vi "rs3_decode_streams2.vi"(0 "Stream profile array":T2(array[cluster])=[{"ID"=42, "Profile"=521622968, "fps"=25, "RS Stream"=0, "RS Format"=0, "index"=2, "width"=1920, "height"=1080, "ppx"=0.0, "ppy"=0.0, "fx"=0.0, "fy"=0.0, "model"=0}, {"ID"=41, "Profile"=521634232, "fps"=25, "RS Stream"=0, "RS Format"=0, "index"=1, "width"=1920, "height"=1080, "ppx"=0.0, "ppy"=0.0, "fx"=0.0, "fy"=0.0, "model"=0}, {"ID"=42, "Profile"=521608632, "fps"=25, "RS Stream"=0, "RS Format"=0, "index"=2, "width"=1920, "height"=1080, "ppx"=951.85925, "ppy"=556.0496, "fx"=1428.9095, "fy"=1428.9095, "model"=4}, {"ID"=41, "Profile"=521617080, "fps"=25, "RS Stream"=0, "RS Format"=0, "index"=1, "width"=1920, "height"=1080, "ppx"=951.85925, "ppy"=556.0496, "fx"=1428.9095, "fy"=1428.9095, "model"=4}, {"ID"=41, "Profile"=521619128, "fps"=15, "RS Stream"=0, "RS Format"=0, "index"=1, "width"=1920, "height"=1080, "ppx"=0.0, "ppy"=0.0, "fx"=0.0, "fy"=0.0, "model"=0}, {"ID"=42, "Profile"=521623224, "fps"=15, "RS Stream"=0, "RS Format"=0, "index"=2, "width"=1920, "height"=1080, "ppx"=0.0, "ppy"=0.0, "fx"=0.0, "fy"=0.0, "model"=0}, {"ID"=42, "Profile"=521628088, "fps"=15, "RS Stream"=0, "RS Format"=0, "index"=2, "width"=1920, "height"=1080, "ppx"=951.85925, "ppy"=556.0496, "fx"=1428.9095, "fy"=1428.9095, "model"=4}, {"ID"=41, "Profile"=521627576, "fps"=15, "RS Stream"=0, "RS Format"=0, "index"=1, "width"=1920, "height"=1080, "ppx"=951.85925, "ppy"=556.0496, "fx"=1428.9095, "fy"=1428.9095, "model"=4}, {"ID"=41, "Profile"=521612728, "fps"=30, "RS Stream"=0, "RS Format"=0, "index"=0, "width"=1280, "height"=720, "ppx"=634.5728, "ppy"=370.69974, "fx"=952.6064, "fy"=952.6064, "model"=4}, {"ID"=41, "Profile"=521610424, "fps"=30, "RS Stream"=0, "RS Format"=0, "index"=0, "width"=1280, "height"=720, "ppx"=0.0, "ppy"=0.0, "fx"=0.0, "fy"=0.0, "model"=0}, {"ID"=42, "Profile"=521615544, "fps"=30, "RS Stream"=0, "RS Format"=0, "index"=2, "width"=1280, "height"=720, "ppx"=634.5728, "ppy"=370.69974, "fx"=952.6064, "fy"=952.6064, "model"=4}, {"ID"=41, "Profile"=521320344, "fps"=30, "RS Stream"=0, "RS Format"=0, "index"=1, "width"=1280, "height"=720, "ppx"=634.5728, "ppy"=370.69974, "fx"=952.6064, "fy"=952.6064, "model"=4}, {"ID"=41, "Profile"=521614520, "fps"=30, "RS Stream"=0, "RS Format"=0, "index"=0, "width"=1280, "height"=720, "ppx"=634.5728, "ppy"=370.69974, "fx"=952.6064, "fy"=952.6064, "model"=4}, {"ID"=41, "Profile"=521605816, "fps"=30, "RS Stream"=0, "RS Format"=0, "index"=0, "width"=1280, "height"=720, "ppx"=634.5728, "ppy"=370.69974, "fx"=952.6064, "fy"=952.6064, "model"=4}, {"ID"=41, "Profile"=521607608, "fps"=30, "RS Stream"=0, "RS Format"=0, "index"=0, "width"=1280, "height"=720, "ppx"=634.5728, "ppy"=370.69974, "fx"=952.6064, "fy"=952.6064, "model"=4}, {"ID"=41, "Profile"=521605560, "fps"=30, "RS Stream"=0, "RS Format"=0, "index"=0, "width"=1280, "height"=720, "ppx"=634.5728, "ppy"=370.69974, "fx"=952.6064, "fy"=952.6064, "model"=4}, {"ID"=41, "Profile"=521609912, "fps"=15, "RS Stream"=0, "RS Format"=0, "index"=0, "width"=1280, "height"=720, "ppx"=634.5728, "ppy"=370.69974, "fx"=952.6064, "fy"=952.6064, "model"=4}, {"ID"=41, "Profile"=521606584, "fps"=15, "RS Stream"=0, "RS Format"=0, "index"=0, "width"=1280, "height"=720, "ppx"=0.0, "ppy"=0.0, "fx"=0.0, "fy"=0.0, "model"=0}, {"ID"=41, "Profile"=521310872, "fps"=15, "RS Stream"=0, "RS Format"=0, "index"=1, "width"=1280, "height"=720, "ppx"=634.5728, "ppy"=370.69974, "fx"=952.6064, "fy"=952.6064, "model"=4}, {"ID"=42, "Profile"=521616824, "fps"=15, "RS Stream"=0, "RS Format"=0, "index"=2, "width"=1280, "height"=720, "ppx"=634.5728, "ppy"=370.69974, "fx"=952.6064, "fy"=952.6064, "model"=4}, {"ID"=41, "Profile"=521604024, "fps"=15, "RS Stream"=0, "RS Format"=0, "index"=0, "width"=1280, "height"=720, "ppx"=634.5728, "ppy"=370.69974, "fx"=952.6064, "fy"=952.6064, "model"=4}, {"ID"=41, "Profile"=521612984, "fps"=15, "RS Stream"=0, "RS Format"=0, "index"=0, "width"=1280, "height"=720, "ppx"=634.5728, "ppy"=370.69974, "fx"=952.6064, "fy"=952.6064, "model"=4}, {"ID"=41, "Profile"=521610168, "fps"=15, "RS Stream"=0, "RS Format"=0, "index"=0, "width"=1280, "height"=720, "ppx"=634.5728, "ppy"=370.69974, "fx"=952.6064, "fy"=952.6064, "model"=4}, {"ID"=41, "Profile"=521604536, "fps"=15, "RS Stream"=0, "RS Format"=0, "index"=0, "width"=1280, "height"=720, "ppx"=634.5728, "ppy"=370.69974, "fx"=952.6064, "fy"=952.6064, "model"=4}, {"ID"=41, "Profile"=521617848, "fps"=6, "RS Stream"=0, "RS Format"=0, "index"=0, "width"=1280, "height"=720, "ppx"=634.5728, "ppy"=370.69974, "fx"=952.6064, "fy"=952.6064, "model"=4}, {"ID"=41, "Profile"=521613752, "fps"=6, "RS Stream"=0, "RS Format"=0, "index"=0, "width"=1280, "height"=720, "ppx"=0.0, "ppy"=0.0, "fx"=0.0, "fy"=0.0, "model"=0}, {"ID"=41, "Profile"=521320600, "fps"=6, "RS Stream"=0, "RS Format"=0, "index"=1, "width"=1280, "height"=720, "ppx"=634.5728, "ppy"=370.69974, "fx"=952.6064, "fy"=952.6064, "model"=4}, {"ID"=42, "Profile"=521608888, "fps"=6, "RS Stream"=0, "RS Format"=0, "index"=2, "width"=1280, "height"=720, "ppx"=634.5728, "ppy"=370.69974, "fx"=952.6064, "fy"=952.6064, "model"=4}, {"ID"=41, "Profile"=521613240, "fps"=6, "RS Stream"=0, "RS Format"=0, "index"=0, "width"=1280, "height"=720, "ppx"=634.5728, "ppy"=370.69974, "fx"=952.6064, "fy"=952.6064, "model"=4}, {"ID"=41, "Profile"=521611704, "fps"=6, "RS Stream"=0, "RS Format"=0, "index"=0, "width"=1280, "height"=720, "ppx"=634.5728, "ppy"=370.69974, "fx"=952.6064, "fy"=952.6064, "model"=4}, {"ID"=41, "Profile"=521601720, "fps"=6, "RS Stream"=0, "RS Format"=0, "index"=0, "width"=1280, "height"=720, "ppx"=634.5728, "ppy"=370.69974, "fx"=952.6064, "fy"=952.6064, "model"=4}, {"ID"=41, "Profile"=521617336, "fps"=6, "RS Stream"=0, "RS Format"=0, "index"=0, "width"=1280, "height"=720, "ppx"=634.5728, "ppy"=370.69974, "fx"=952.6064, "fy"=952.6064, "model"=4}, {"ID"=41, "Profile"=521622712, "fps"=25, "RS Stream"=0, "RS Format"=0, "index"=1, "width"=960, "height"=540, "ppx"=0.0, "ppy"=0.0, "fx"=0.0, "fy"=0.0, "model"=0}, {"ID"=42, "Profile"=521633976, "fps"=25, "RS Stream"=0, "RS Format"=0, "index"=2, "width"=960, "height"=540, "ppx"=0.0, "ppy"=0.0, "fx"=0.0, "fy"=0.0, "model"=0}, {"ID"=42, "Profile"=521624504, "fps"=15, "RS Stream"=0, "RS Format"=0, "index"=2, "width"=960, "height"=540, "ppx"=0.0, "ppy"=0.0, "fx"=0.0, "fy"=0.0, "model"=0}, {"ID"=41, "Profile"=521622456, "fps"=15, "RS Stream"=0, "RS Format"=0, "index"=1, "width"=960, "height"=540, "ppx"=0.0, "ppy"=0.0, "fx"=0.0, "fy"=0.0, "model"=0}, {"ID"=41, "Profile"=521352856, "fps"=90, "RS Stream"=0, "RS Format"=0, "index"=0, "width"=848, "height"=480, "ppx"=420.38187, "ppy"=247.13316, "fx"=635.0709, "fy"=635.0709, "model"=4}, {"ID"=41, "Profile"=521351320, "fps"=90, "RS Stream"=0, "RS Format"=0, "index"=0, "width"=848, "height"=480, "ppx"=0.0, "ppy"=0.0, "fx"=0.0, "fy"=0.0, "model"=0}, {"ID"=41, "Profile"=521306776, "fps"=90, "RS Stream"=0, "RS Format"=0, "index"=1, "width"=848, "height"=480, "ppx"=420.38187, "ppy"=247.13316, "fx"=635.0709, "fy"=635.0709, "model"=4}, {"ID"=42, "Profile"=521614776, "fps"=90, "RS Stream"=0, "RS Format"=0, "index"=2, "width"=848, "height"=480, "ppx"=420.38187, "ppy"=247.13316, "fx"=635.0709, "fy"=635.0709, "model"=4}, {"ID"=41, "Profile"=521353624, "fps"=90, "RS Stream"=0, "RS Format"=0, "index"=0, "width"=848, "height"=480, "ppx"=420.38187, "ppy"=247.13316, "fx"=635.0709, "fy"=635.0709, "model"=4}, {"ID"=41, "Profile"=521339544, "fps"=90, "RS Stream"=0, "RS Format"=0, "index"=0, "width"=848, "height"=480, "ppx"=420.38187, "ppy"=247.13316, "fx"=635.0709, "fy"=635.0709, "model"=4}, {"ID"=41, "Profile"=521353368, "fps"=90, "RS Stream"=0, "RS Format"=0, "index"=0, "width"=848, "height"=480, "ppx"=420.38187, "ppy"=247.13316, "fx"=635.0709, "fy"=635.0709, "model"=4}, {"ID"=41, "Profile"=521351064, "fps"=90, "RS Stream"=0, "RS Format"=0, "index"=0, "width"=848, "height"=480, "ppx"=420.38187, "ppy"=247.13316, "fx"=635.0709, "fy"=635.0709, "model"=4}, {"ID"=41, "Profile"=521342104, "fps"=60, "RS Stream"=0, "RS Format"=0, "index"=0, "width"=848, "height"=480, "ppx"=420.38187, "ppy"=247.13316, "fx"=635.0709, "fy"=635.0709, "model"=4}, {"ID"=41, "Profile"=521341848, "fps"=60, "RS Stream"=0, "RS Format"=0, "index"=0, "width"=848, "height"=480, "ppx"=0.0, "ppy"=0.0, "fx"=0.0, "fy"=0.0, "model"=0}, {"ID"=42, "Profile"=521611960, "fps"=60, "RS Stream"=0, "RS Format"=0, "index"=2, "width"=848, "height"=480, "ppx"=420.38187, "ppy"=247.13316, "fx"=635.0709, "fy"=635.0709, "model"=4}, {"ID"=41, "Profile"=521310360, "fps"=60, "RS Stream"=0, "RS Format"=0, "index"=1, "width"=848, "height"=480, "ppx"=420.38187, "ppy"=247.13316, "fx"=635.0709, "fy"=635.0709, "model"=4}, {"ID"=41, "Profile"=521343384, "fps"=60, "RS Stream"=0, "RS Format"=0, "index"=0, "width"=848, "height"=480, "ppx"=420.38187, "ppy"=247.13316, "fx"=635.0709, "fy"=635.0709, "model"=4}, {"ID"=41, "Profile"=521342360, "fps"=60, "RS Stream"=0, "RS Format"=0, "index"=0, "width"=848, "height"=480, "ppx"=420.38187, "ppy"=247.13316, "fx"=635.0709, "fy"=635.0709, "model"=4}, {"ID"=41, "Profile"=521342616, "fps"=60, "RS Stream"=0, "RS Format"=0, "index"=0, "width"=848, "height"=480, "ppx"=420.38187, "ppy"=247.13316, "fx"=635.0709, "fy"=635.0709, "model"=4}, {"ID"=41, "Profile"=521354136, "fps"=60, "RS Stream"=0, "RS Format"=0, "index"=0, "width"=848, "height"=480, "ppx"=420.38187, "ppy"=247.13316, "fx"=635.0709, "fy"=635.0709, "model"=4}, {"ID"=41, "Profile"=521616056, "fps"=30, "RS Stream"=0, "RS Format"=0, "index"=0, "width"=848, "height"=480, "ppx"=420.38187, "ppy"=247.13316, "fx"=635.0709, "fy"=635.0709, "model"=4}, {"ID"=41, "Profile"=514733800, "fps"=30, "RS Stream"=0, "RS Format"=0, "index"=0, "width"=848, "height"=480, "ppx"=0.0, "ppy"=0.0, "fx"=0.0, "fy"=0.0, "model"=0}, {"ID"=42, "Profile"=521609144, "fps"=30, "RS Stream"=0, "RS Format"=0, "index"=2, "width"=848, "height"=480, "ppx"=420.38187, "ppy"=247.13316, "fx"=635.0709, "fy"=635.0709, "model"=4}, {"ID"=41, "Profile"=521310616, "fps"=30, "RS Stream"=0, "RS Format"=0, "index"=1, "width"=848, "height"=480, "ppx"=420.38187, "ppy"=247.13316, "fx"=635.0709, "fy"=635.0709, "model"=4}, {"ID"=41, "Profile"=521606840, "fps"=30, "RS Stream"=0, "RS Format"=0, "index"=0, "width"=848, "height"=480, "ppx"=420.38187, "ppy"=247.13316, "fx"=635.0709, "fy"=635.0709, "model"=4}, {"ID"=41, "Profile"=521603256, "fps"=30, "RS Stream"=0, "RS Format"=0, "index"=0, "width"=848, "height"=480, "ppx"=420.38187, "ppy"=247.13316, "fx"=635.0709, "fy"=635.0709, "model"=4}, {"ID"=41, "Profile"=521612472, "fps"=30, "RS Stream"=0, "RS Format"=0, "index"=0, "width"=848, "height"=480, "ppx"=420.38187, "ppy"=247.13316, "fx"=635.0709, "fy"=635.0709, "model"=4}, {"ID"=41, "Profile"=521343640, "fps"=30, "RS Stream"=0, "RS Format"=0, "index"=0, "width"=848, "height"=480, "ppx"=420.38187, "ppy"=247.13316, "fx"=635.0709, "fy"=635.0709, "model"=4}, {"ID"=41, "Profile"=521609400, "fps"=15, "RS Stream"=0, "RS Format"=0, "index"=0, "width"=848, "height"=480, "ppx"=420.38187, "ppy"=247.13316, "fx"=635.0709, "fy"=635.0709, "model"=4}, {"ID"=41, "Profile"=521606328, "fps"=15, "RS Stream"=0, "RS Format"=0, "index"=0, "width"=848, "height"=480, "ppx"=0.0, "ppy"=0.0, "fx"=0.0, "fy"=0.0, "model"=0}, {"ID"=41, "Profile"=521317272, "fps"=15, "RS Stream"=0, "RS Format"=0, "index"=1, "width"=848, "height"=480, "ppx"=420.38187, "ppy"=247.13316, "fx"=635.0709, "fy"=635.0709, "model"=4}, {"ID"=42, "Profile"=521615288, "fps"=15, "RS Stream"=0, "RS Format"=0, "index"=2, "width"=848, "height"=480, "ppx"=420.38187, "ppy"=247.13316, "fx"=635.0709, "fy"=635.0709, "model"=4}, {"ID"=41, "Profile"=521603512, "fps"=15, "RS Stream"=0, "RS Format"=0, "index"=0, "width"=848, "height"=480, "ppx"=420.38187, "ppy"=247.13316, "fx"=635.0709, "fy"=635.0709, "model"=4}, {"ID"=41, "Profile"=521602744, "fps"=15, "RS Stream"=0, "RS Format"=0, "index"=0, "width"=848, "height"=480, "ppx"=420.38187, "ppy"=247.13316, "fx"=635.0709, "fy"=635.0709, "model"=4}, {"ID"=41, "Profile"=521607096, "fps"=15, "RS Stream"=0, "RS Format"=0, "index"=0, "width"=848, "height"=480, "ppx"=420.38187, "ppy"=247.13316, "fx"=635.0709, "fy"=635.0709, "model"=4}, {"ID"=41, "Profile"=521617592, "fps"=15, "RS Stream"=0, "RS Format"=0, "index"=0, "width"=848, "height"=480, "ppx"=420.38187, "ppy"=247.13316, "fx"=635.0709, "fy"=635.0709, "model"=4}, {"ID"=41, "Profile"=521603768, "fps"=6, "RS Stream"=0, "RS Format"=0, "index"=0, "width"=848, "height"=480, "ppx"=420.38187, "ppy"=247.13316, "fx"=635.0709, "fy"=635.0709, "model"=4}, {"ID"=41, "Profile"=521604280, "fps"=6, "RS Stream"=0, "RS Format"=0, "index"=0, "width"=848, "height"=480, "ppx"=0.0, "ppy"=0.0, "fx"=0.0, "fy"=0.0, "model"=0}, {"ID"=42, "Profile"=521616568, "fps"=6, "RS Stream"=0, "RS Format"=0, "index"=2, "width"=848, "height"=480, "ppx"=420.38187, "ppy"=247.13316, "fx"=635.0709, "fy"=635.0709, "model"=4}, {"ID"=41, "Profile"=521315992, "fps"=6, "RS Stream"=0, "RS Format"=0, "index"=1, "width"=848, "height"=480, "ppx"=420.38187, "ppy"=247.13316, "fx"=635.0709, "fy"=635.0709, "model"=4}, {"ID"=41, "Profile"=521607864, "fps"=6, "RS Stream"=0, "RS Format"=0, "index"=0, "width"=848, "height"=480, "ppx"=420.38187, "ppy"=247.13316, "fx"=635.0709, "fy"=635.0709, "model"=4}, {"ID"=41, "Profile"=521616312, "fps"=6, "RS Stream"=0, "RS Format"=0, "index"=0, "width"=848, "height"=480, "ppx"=420.38187, "ppy"=247.13316, "fx"=635.0709, "fy"=635.0709, "model"=4}, {"ID"=41, "Profile"=521615800, "fps"=6, "RS Stream"=0, "RS Format"=0, "index"=0, "width"=848, "height"=480, "ppx"=420.38187, "ppy"=247.13316, "fx"=635.0709, "fy"=635.0709, "model"=4}, {"ID"=41, "Profile"=521610680, "fps"=6, "RS Stream"=0, "RS Format"=0, "index"=0, "width"=848, "height"=480, "ppx"=420.38187, "ppy"=247.13316, "fx"=635.0709, "fy"=635.0709, "model"=4}, {"ID"=41, "Profile"=521348504, "fps"=90, "RS Stream"=0, "RS Format"=0, "index"=0, "width"=640, "height"=480, "ppx"=316.38187, "ppy"=247.13316, "fx"=635.0709, "fy"=635.0709, "model"=4}, {"ID"=41, "Profile"=521354904, "fps"=90, "RS Stream"=0, "RS Format"=0, "index"=0, "width"=640, "height"=480, "ppx"=0.0, "ppy"=0.0, "fx"=0.0, "fy"=0.0, "model"=0}, {"ID"=42, "Profile"=521605304, "fps"=90, "RS Stream"=0, "RS Format"=0, "index"=2, "width"=640, "height"=480, "ppx"=316.38187, "ppy"=247.13316, "fx"=635.0709, "fy"=635.0709, "model"=4}, {"ID"=41, "Profile"=521322648, "fps"=90, "RS Stream"=0, "RS Format"=0, "index"=1, "width"=640, "height"=480, "ppx"=316.38187, "ppy"=247.13316, "fx"=635.0709, "fy"=635.0709, "model"=4}, {"ID"=41, "Profile"=521340056, "fps"=90, "RS Stream"=0, "RS Format"=0, "index"=0, "width"=640, "height"=480, "ppx"=316.38187, "ppy"=247.13316, "fx"=635.0709, "fy"=635.0709, "model"=4}, {"ID"=41, "Profile"=521355672, "fps"=90, "RS Stream"=0, "RS Format"=0, "index"=0, "width"=640, "height"=480, "ppx"=316.38187, "ppy"=247.13316, "fx"=635.0709, "fy"=635.0709, "model"=4}, {"ID"=41, "Profile"=521352088, "fps"=90, "RS Stream"=0, "RS Format"=0, "index"=0, "width"=640, "height"=480, "ppx"=316.38187, "ppy"=247.13316, "fx"=635.0709, "fy"=635.0709, "model"=4}, {"ID"=41, "Profile"=521351576, "fps"=90, "RS Stream"=0, "RS Format"=0, "index"=0, "width"=640, "height"=480, "ppx"=316.38187, "ppy"=247.13316, "fx"=635.0709, "fy"=635.0709, "model"=4}, {"ID"=41, "Profile"=521352344, "fps"=60, "RS Stream"=0, "RS Format"=0, "index"=0, "width"=640, "height"=480, "ppx"=316.38187, "ppy"=247.13316, "fx"=635.0709, "fy"=635.0709, "model"=4}, {"ID"=41, "Profile"=521354648, "fps"=60, "RS Stream"=0, "RS Format"=0, "index"=0, "width"=640, "height"=480, "ppx"=0.0, "ppy"=0.0, "fx"=0.0, "fy"=0.0, "model"=0}, {"ID"=41, "Profile"=521320088, "fps"=60, "RS Stream"=0, "RS Format"=0, "index"=1, "width"=640, "height"=480, "ppx"=316.38187, "ppy"=247.13316, "fx"=635.0709, "fy"=635.0709, "model"=4}, {"ID"=42, "Profile"=521615032, "fps"=60, "RS Stream"=0, "RS Format"=0, "index"=2, "width"=640, "height"=480, "ppx"=316.38187, "ppy"=247.13316, "fx"=635.0709, "fy"=635.0709, "model"=4}, {"ID"=41, "Profile"=521340312, "fps"=60, "RS Stream"=0, "RS Format"=0, "index"=0, "width"=640, "height"=480, "ppx"=316.38187, "ppy"=247.13316, "fx"=635.0709, "fy"=635.0709, "model"=4}, {"ID"=41, "Profile"=521342872, "fps"=60, "RS Stream"=0, "RS Format"=0, "index"=0, "width"=640, "height"=480, "ppx"=316.38187, "ppy"=247.13316, "fx"=635.0709, "fy"=635.0709, "model"=4}, {"ID"=41, "Profile"=521346200, "fps"=60, "RS Stream"=0, "RS Format"=0, "index"=0, "width"=640, "height"=480, "ppx"=316.38187, "ppy"=247.13316, "fx"=635.0709, "fy"=635.0709, "model"=4}, {"ID"=41, "Profile"=521345944, "fps"=60, "RS Stream"=0, "RS Format"=0, "index"=0, "width"=640, "height"=480, "ppx"=316.38187, "ppy"=247.13316, "fx"=635.0709, "fy"=635.0709, "model"=4}, {"ID"=41, "Profile"=521344408, "fps"=30, "RS Stream"=0, "RS Format"=0, "index"=0, "width"=640, "height"=480, "ppx"=316.38187, "ppy"=247.13316, "fx"=635.0709, "fy"=635.0709, "model"=4}, {"ID"=41, "Profile"=521348248, "fps"=30, "RS Stream"=0, "RS Format"=0, "index"=0, "width"=640, "height"=480, "ppx"=0.0, "ppy"=0.0, "fx"=0.0, "fy"=0.0, "model"=0}, {"ID"=41, "Profile"=521309592, "fps"=30, "RS Stream"=0, "RS Format"=0, "index"=1, "width"=640, "height"=480, "ppx"=316.38187, "ppy"=247.13316, "fx"=635.0709, "fy"=635.0709, "model"=4}, {"ID"=42, "Profile"=521607352, "fps"=30, "RS Stream"=0, "RS Format"=0, "index"=2, "width"=640, "height"=480, "ppx"=316.38187, "ppy"=247.13316, "fx"=635.0709, "fy"=635.0709, "model"=4}, {"ID"=41, "Profile"=521352600, "fps"=30, "RS Stream"=0, "RS Format"=0, "index"=0, "width"=640, "height"=480, "ppx"=316.38187, "ppy"=247.13316, "fx"=635.0709, "fy"=635.0709, "model"=4}, {"ID"=41, "Profile"=521344664, "fps"=30, "RS Stream"=0, "RS Format"=0, "index"=0, "width"=640, "height"=480, "ppx"=316.38187, "ppy"=247.13316, "fx"=635.0709, "fy"=635.0709, "model"=4}, {"ID"=41, "Profile"=521344920, "fps"=30, "RS Stream"=0, "RS Format"=0, "index"=0, "width"=640, "height"=480, "ppx"=316.38187, "ppy"=247.13316, "fx"=635.0709, "fy"=635.0709, "model"=4}, {"ID"=41, "Profile"=521350296, "fps"=30, "RS Stream"=0, "RS Format"=0, "index"=0, "width"=640, "height"=480, "ppx"=316.38187, "ppy"=247.13316, "fx"=635.0709, "fy"=635.0709, "model"=4}, {"ID"=41, "Profile"=521355160, "fps"=15, "RS Stream"=0, "RS Format"=0, "index"=0, "width"=640, "height"=480, "ppx"=316.38187, "ppy"=247.13316, "fx"=635.0709, "fy"=635.0709, "model"=4}, {"ID"=41, "Profile"=521341592, "fps"=15, "RS Stream"=0, "RS Format"=0, "index"=0, "width"=640, "height"=480, "ppx"=0.0, "ppy"=0.0, "fx"=0.0, "fy"=0.0, "model"=0}, {"ID"=41, "Profile"=521321368, "fps"=15, "RS Stream"=0, "RS Format"=0, "index"=1, "width"=640, "height"=480, "ppx"=316.38187, "ppy"=247.13316, "fx"=635.0709, "fy"=635.0709, "model"=4}, {"ID"=42, "Profile"=521608120, "fps"=15, "RS Stream"=0, "RS Format"=0, "index"=2, "width"=640, "height"=480, "ppx"=316.38187, "ppy"=247.13316, "fx"=635.0709, "fy"=635.0709, "model"=4}, {"ID"=41, "Profile"=521346968, "fps"=15, "RS Stream"=0, "RS Format"=0, "index"=0, "width"=640, "height"=480, "ppx"=316.38187, "ppy"=247.13316, "fx"=635.0709, "fy"=635.0709, "model"=4}, {"ID"=41, "Profile"=521348760, "fps"=15, "RS Stream"=0, "RS Format"=0, "index"=0, "width"=640, "height"=480, "ppx"=316.38187, "ppy"=247.13316, "fx"=635.0709, "fy"=635.0709, "model"=4}, {"ID"=41, "Profile"=521339800, "fps"=15, "RS Stream"=0, "RS Format"=0, "index"=0, "width"=640, "height"=480, "ppx"=316.38187, "ppy"=247.13316, "fx"=635.0709, "fy"=635.0709, "model"=4}, {"ID"=41, "Profile"=521350808, "fps"=15, "RS Stream"=0, "RS Format"=0, "index"=0, "width"=640, "height"=480, "ppx"=316.38187, "ppy"=247.13316, "fx"=635.0709, "fy"=635.0709, "model"=4}, {"ID"=41, "Profile"=521349016, "fps"=6, "RS Stream"=0, "RS Format"=0, "index"=0, "width"=640, "height"=480, "ppx"=316.38187, "ppy"=247.13316, "fx"=635.0709, "fy"=635.0709, "model"=4}, {"ID"=41, "Profile"=521346456, "fps"=6, "RS Stream"=0, "RS Format"=0, "index"=0, "width"=640, "height"=480, "ppx"=0.0, "ppy"=0.0, "fx"=0.0, "fy"=0.0, "model"=0}, {"ID"=42, "Profile"=521608376, "fps"=6, "RS Stream"=0, "RS Format"=0, "index"=2, "width"=640, "height"=480, "ppx"=316.38187, "ppy"=247.13316, "fx"=635.0709, "fy"=635.0709, "model"=4}, {"ID"=41, "Profile"=521313176, "fps"=6, "RS Stream"=0, "RS Format"=0, "index"=1, "width"=640, "height"=480, "ppx"=316.38187, "ppy"=247.13316, "fx"=635.0709, "fy"=635.0709, "model"=4}, {"ID"=41, "Profile"=521343128, "fps"=6, "RS Stream"=0, "RS Format"=0, "index"=0, "width"=640, "height"=480, "ppx"=316.38187, "ppy"=247.13316, "fx"=635.0709, "fy"=635.0709, "model"=4}, {"ID"=41, "Profile"=521349528, "fps"=6, "RS Stream"=0, "RS Format"=0, "index"=0, "width"=640, "height"=480, "ppx"=316.38187, "ppy"=247.13316, "fx"=635.0709, "fy"=635.0709, "model"=4}, {"ID"=41, "Profile"=521355416, "fps"=6, "RS Stream"=0, "RS Format"=0, "index"=0, "width"=640, "height"=480, "ppx"=316.38187, "ppy"=247.13316, "fx"=635.0709, "fy"=635.0709, "model"=4}, {"ID"=41, "Profile"=521349272, "fps"=6, "RS Stream"=0, "RS Format"=0, "index"=0, "width"=640, "height"=480, "ppx"=316.38187, "ppy"=247.13316, "fx"=635.0709, "fy"=635.0709, "model"=4}, {"ID"=41, "Profile"=521330840, "fps"=90, "RS Stream"=0, "RS Format"=0, "index"=0, "width"=640, "height"=360, "ppx"=317.2864, "ppy"=185.34987, "fx"=476.3032, "fy"=476.3032, "model"=4}, {"ID"=41, "Profile"=521330584, "fps"=90, "RS Stream"=0, "RS Format"=0, "index"=0, "width"=640, "height"=360, "ppx"=0.0, "ppy"=0.0, "fx"=0.0, "fy"=0.0, "model"=0}, {"ID"=41, "Profile"=521318296, "fps"=90, "RS Stream"=0, "RS Format"=0, "index"=1, "width"=640, "height"=360, "ppx"=317.2864, "ppy"=185.34987, "fx"=476.3032, "fy"=476.3032, "model"=4}, {"ID"=42, "Profile"=521609656, "fps"=90, "RS Stream"=0, "RS Format"=0, "index"=2, "width"=640, "height"=360, "ppx"=317.2864, "ppy"=185.34987, "fx"=476.3032, "fy"=476.3032, "model"=4}, {"ID"=41, "Profile"=521332120, "fps"=90, "RS Stream"=0, "RS Format"=0, "index"=0, "width"=640, "height"=360, "ppx"=317.2864, "ppy"=185.34987, "fx"=476.3032, "fy"=476.3032, "model"=4}, {"ID"=41, "Profile"=521331608, "fps"=90, "RS Stream"=0, "RS Format"=0, "index"=0, "width"=640, "height"=360, "ppx"=317.2864, "ppy"=185.34987, "fx"=476.3032, "fy"=476.3032, "model"=4}, {"ID"=41, "Profile"=521331864, "fps"=90, "RS Stream"=0, "RS Format"=0, "index"=0, "width"=640, "height"=360, "ppx"=317.2864, "ppy"=185.34987, "fx"=476.3032, "fy"=476.3032, "model"=4}, {"ID"=41, "Profile"=521326744, "fps"=90, "RS Stream"=0, "RS Format"=0, "index"=0, "width"=640, "height"=360, "ppx"=317.2864, "ppy"=185.34987, "fx"=476.3032, "fy"=476.3032, "model"=4}, {"ID"=41, "Profile"=521333912, "fps"=60, "RS Stream"=0, "RS Format"=0, "index"=0, "width"=640, "height"=360, "ppx"=317.2864, "ppy"=185.34987, "fx"=476.3032, "fy"=476.3032, "model"=4}, {"ID"=41, "Profile"=521333144, "fps"=60, "RS Stream"=0, "RS Format"=0, "index"=0, "width"=640, "height"=360, "ppx"=0.0, "ppy"=0.0, "fx"=0.0, "fy"=0.0, "model"=0}, {"ID"=42, "Profile"=521606072, "fps"=60, "RS Stream"=0, "RS Format"=0, "index"=2, "width"=640, "height"=360, "ppx"=317.2864, "ppy"=185.34987, "fx"=476.3032, "fy"=476.3032, "model"=4}, {"ID"=41, "Profile"=521321112, "fps"=60, "RS Stream"=0, "RS Format"=0, "index"=1, "width"=640, "height"=360, "ppx"=317.2864, "ppy"=185.34987, "fx"=476.3032, "fy"=476.3032, "model"=4}, {"ID"=41, "Profile"=521340824, "fps"=60, "RS Stream"=0, "RS Format"=0, "index"=0, "width"=640, "height"=360, "ppx"=317.2864, "ppy"=185.34987, "fx"=476.3032, "fy"=476.3032, "model"=4}, {"ID"=41, "Profile"=521353880, "fps"=60, "RS Stream"=0, "RS Format"=0, "index"=0, "width"=640, "height"=360, "ppx"=317.2864, "ppy"=185.34987, "fx"=476.3032, "fy"=476.3032, "model"=4}, {"ID"=41, "Profile"=521350552, "fps"=60, "RS Stream"=0, "RS Format"=0, "index"=0, "width"=640, "height"=360, "ppx"=317.2864, "ppy"=185.34987, "fx"=476.3032, "fy"=476.3032, "model"=4}, {"ID"=41, "Profile"=521332888, "fps"=60, "RS Stream"=0, "RS Format"=0, "index"=0, "width"=640, "height"=360, "ppx"=317.2864, "ppy"=185.34987, "fx"=476.3032, "fy"=476.3032, "model"=4}, {"ID"=41, "Profile"=521347224, "fps"=30, "RS Stream"=0, "RS Format"=0, "index"=0, "width"=640, "height"=360, "ppx"=317.2864, "ppy"=185.34987, "fx"=476.3032, "fy"=476.3032, "model"=4}, {"ID"=41, "Profile"=521349784, "fps"=30, "RS Stream"=0, "RS Format"=0, "index"=0, "width"=640, "height"=360, "ppx"=0.0, "ppy"=0.0, "fx"=0.0, "fy"=0.0, "model"=0}, {"ID"=42, "Profile"=521604792, "fps"=30, "RS Stream"=0, "RS Format"=0, "index"=2, "width"=640, "height"=360, "ppx"=317.2864, "ppy"=185.34987, "fx"=476.3032, "fy"=476.3032, "model"=4}, {"ID"=41, "Profile"=521319064, "fps"=30, "RS Stream"=0, "RS Format"=0, "index"=1, "width"=640, "height"=360, "ppx"=317.2864, "ppy"=185.34987, "fx"=476.3032, "fy"=476.3032, "model"=4}, {"ID"=41, "Profile"=521351832, "fps"=30, "RS Stream"=0, "RS Format"=0, "index"=0, "width"=640, "height"=360, "ppx"=317.2864, "ppy"=185.34987, "fx"=476.3032, "fy"=476.3032, "model"=4}, {"ID"=41, "Profile"=521347480, "fps"=30, "RS Stream"=0, "RS Format"=0, "index"=0, "width"=640, "height"=360, "ppx"=317.2864, "ppy"=185.34987, "fx"=476.3032, "fy"=476.3032, "model"=4}, {"ID"=41, "Profile"=521350040, "fps"=30, "RS Stream"=0, "RS Format"=0, "index"=0, "width"=640, "height"=360, "ppx"=317.2864, "ppy"=185.34987, "fx"=476.3032, "fy"=476.3032, "model"=4}, {"ID"=41, "Profile"=521345432, "fps"=30, "RS Stream"=0, "RS Format"=0, "index"=0, "width"=640, "height"=360, "ppx"=317.2864, "ppy"=185.34987, "fx"=476.3032, "fy"=476.3032, "model"=4}, {"ID"=41, "Profile"=521343896, "fps"=15, "RS Stream"=0, "RS Format"=0, "index"=0, "width"=640, "height"=360, "ppx"=317.2864, "ppy"=185.34987, "fx"=476.3032, "fy"=476.3032, "model"=4}, {"ID"=41, "Profile"=521340568, "fps"=15, "RS Stream"=0, "RS Format"=0, "index"=0, "width"=640, "height"=360, "ppx"=0.0, "ppy"=0.0, "fx"=0.0, "fy"=0.0, "model"=0}, {"ID"=41, "Profile"=521319320, "fps"=15, "RS Stream"=0, "RS Format"=0, "index"=1, "width"=640, "height"=360, "ppx"=317.2864, "ppy"=185.34987, "fx"=476.3032, "fy"=476.3032, "model"=4}, {"ID"=42, "Profile"=521613496, "fps"=15, "RS Stream"=0, "RS Format"=0, "index"=2, "width"=640, "height"=360, "ppx"=317.2864, "ppy"=185.34987, "fx"=476.3032, "fy"=476.3032, "model"=4}, {"ID"=41, "Profile"=521347736, "fps"=15, "RS Stream"=0, "RS Format"=0, "index"=0, "width"=640, "height"=360, "ppx"=317.2864, "ppy"=185.34987, "fx"=476.3032, "fy"=476.3032, "model"=4}, {"ID"=41, "Profile"=521345176, "fps"=15, "RS Stream"=0, "RS Format"=0, "index"=0, "width"=640, "height"=360, "ppx"=317.2864, "ppy"=185.34987, "fx"=476.3032, "fy"=476.3032, "model"=4}, {"ID"=41, "Profile"=521345688, "fps"=15, "RS Stream"=0, "RS Format"=0, "index"=0, "width"=640, "height"=360, "ppx"=317.2864, "ppy"=185.34987, "fx"=476.3032, "fy"=476.3032, "model"=4}, {"ID"=41, "Profile"=521347992, "fps"=15, "RS Stream"=0, "RS Format"=0, "index"=0, "width"=640, "height"=360, "ppx"=317.2864, "ppy"=185.34987, "fx"=476.3032, "fy"=476.3032, "model"=4}, {"ID"=41, "Profile"=521354392, "fps"=6, "RS Stream"=0, "RS Format"=0, "index"=0, "width"=640, "height"=360, "ppx"=317.2864, "ppy"=185.34987, "fx"=476.3032, "fy"=476.3032, "model"=4}, {"ID"=41, "Profile"=521341080, "fps"=6, "RS Stream"=0, "RS Format"=0, "index"=0, "width"=640, "height"=360, "ppx"=0.0, "ppy"=0.0, "fx"=0.0, "fy"=0.0, "model"=0}, {"ID"=42, "Profile"=521611448, "fps"=6, "RS Stream"=0, "RS Format"=0, "index"=2, "width"=640, "height"=360, "ppx"=317.2864, "ppy"=185.34987, "fx"=476.3032, "fy"=476.3032, "model"=4}, {"ID"=41, "Profile"=521314200, "fps"=6, "RS Stream"=0, "RS Format"=0, "index"=1, "width"=640, "height"=360, "ppx"=317.2864, "ppy"=185.34987, "fx"=476.3032, "fy"=476.3032, "model"=4}, {"ID"=41, "Profile"=521341336, "fps"=6, "RS Stream"=0, "RS Format"=0, "index"=0, "width"=640, "height"=360, "ppx"=317.2864, "ppy"=185.34987, "fx"=476.3032, "fy"=476.3032, "model"=4}, {"ID"=41, "Profile"=521344152, "fps"=6, "RS Stream"=0, "RS Format"=0, "index"=0, "width"=640, "height"=360, "ppx"=317.2864, "ppy"=185.34987, "fx"=476.3032, "fy"=476.3032, "model"=4}, {"ID"=41, "Profile"=521346712, "fps"=6, "RS Stream"=0, "RS Format"=0, "index"=0, "width"=640, "height"=360, "ppx"=317.2864, "ppy"=185.34987, "fx"=476.3032, "fy"=476.3032, "model"=4}, {"ID"=41, "Profile"=521353112, "fps"=6, "RS Stream"=0, "RS Format"=0, "index"=0, "width"=640, "height"=360, "ppx"=317.2864, "ppy"=185.34987, "fx"=476.3032, "fy"=476.3032, "model"=4}, {"ID"=41, "Profile"=521325720, "fps"=90, "RS Stream"=0, "RS Format"=0, "index"=0, "width"=480, "height"=270, "ppx"=237.96481, "ppy"=139.0124, "fx"=357.2274, "fy"=357.2274, "model"=4}, {"ID"=41, "Profile"=521331096, "fps"=90, "RS Stream"=0, "RS Format"=0, "index"=0, "width"=480, "height"=270, "ppx"=0.0, "ppy"=0.0, "fx"=0.0, "fy"=0.0, "model"=0}, {"ID"=42, "Profile"=521612216, "fps"=90, "RS Stream"=0, "RS Format"=0, "index"=2, "width"=480, "height"=270, "ppx"=237.96481, "ppy"=139.0124, "fx"=357.2274, "fy"=357.2274, "model"=4}, {"ID"=41, "Profile"=521312152, "fps"=90, "RS Stream"=0, "RS Format"=0, "index"=1, "width"=480, "height"=270, "ppx"=237.96481, "ppy"=139.0124, "fx"=357.2274, "fy"=357.2274, "model"=4}, {"ID"=41, "Profile"=521327768, "fps"=90, "RS Stream"=0, "RS Format"=0, "index"=0, "width"=480, "height"=270, "ppx"=237.96481, "ppy"=139.0124, "fx"=357.2274, "fy"=357.2274, "model"=4}, {"ID"=41, "Profile"=521336472, "fps"=90, "RS Stream"=0, "RS Format"=0, "index"=0, "width"=480, "height"=270, "ppx"=237.96481, "ppy"=139.0124, "fx"=357.2274, "fy"=357.2274, "model"=4}, {"ID"=41, "Profile"=521336728, "fps"=90, "RS Stream"=0, "RS Format"=0, "index"=0, "width"=480, "height"=270, "ppx"=237.96481, "ppy"=139.0124, "fx"=357.2274, "fy"=357.2274, "model"=4}, {"ID"=41, "Profile"=521326232, "fps"=90, "RS Stream"=0, "RS Format"=0, "index"=0, "width"=480, "height"=270, "ppx"=237.96481, "ppy"=139.0124, "fx"=357.2274, "fy"=357.2274, "model"=4}, {"ID"=41, "Profile"=521336984, "fps"=60, "RS Stream"=0, "RS Format"=0, "index"=0, "width"=480, "height"=270, "ppx"=237.96481, "ppy"=139.0124, "fx"=357.2274, "fy"=357.2274, "model"=4}, {"ID"=41, "Profile"=521328024, "fps"=60, "RS Stream"=0, "RS Format"=0, "index"=0, "width"=480, "height"=270, "ppx"=0.0, "ppy"=0.0, "fx"=0.0, "fy"=0.0, "model"=0}, {"ID"=41, "Profile"=521322904, "fps"=60, "RS Stream"=0, "RS Format"=0, "index"=1, "width"=480, "height"=270, "ppx"=237.96481, "ppy"=139.0124, "fx"=357.2274, "fy"=357.2274, "model"=4}, {"ID"=42, "Profile"=521603000, "fps"=60, "RS Stream"=0, "RS Format"=0, "index"=2, "width"=480, "height"=270, "ppx"=237.96481, "ppy"=139.0124, "fx"=357.2274, "fy"=357.2274, "model"=4}, {"ID"=41, "Profile"=521338264, "fps"=60, "RS Stream"=0, "RS Format"=0, "index"=0, "width"=480, "height"=270, "ppx"=237.96481, "ppy"=139.0124, "fx"=357.2274, "fy"=357.2274, "model"=4}, {"ID"=41, "Profile"=521337752, "fps"=60, "RS Stream"=0, "RS Format"=0, "index"=0, "width"=480, "height"=270, "ppx"=237.96481, "ppy"=139.0124, "fx"=357.2274, "fy"=357.2274, "model"=4}, {"ID"=41, "Profile"=521323416, "fps"=60, "RS Stream"=0, "RS Format"=0, "index"=0, "width"=480, "height"=270, "ppx"=237.96481, "ppy"=139.0124, "fx"=357.2274, "fy"=357.2274, "model"=4}, {"ID"=41, "Profile"=521337496, "fps"=60, "RS Stream"=0, "RS Format"=0, "index"=0, "width"=480, "height"=270, "ppx"=237.96481, "ppy"=139.0124, "fx"=357.2274, "fy"=357.2274, "model"=4}, {"ID"=41, "Profile"=521329816, "fps"=30, "RS Stream"=0, "RS Format"=0, "index"=0, "width"=480, "height"=270, "ppx"=237.96481, "ppy"=139.0124, "fx"=357.2274, "fy"=357.2274, "model"=4}, {"ID"=41, "Profile"=521328280, "fps"=30, "RS Stream"=0, "RS Format"=0, "index"=0, "width"=480, "height"=270, "ppx"=0.0, "ppy"=0.0, "fx"=0.0, "fy"=0.0, "model"=0}, {"ID"=42, "Profile"=521605048, "fps"=30, "RS Stream"=0, "RS Format"=0, "index"=2, "width"=480, "height"=270, "ppx"=237.96481, "ppy"=139.0124, "fx"=357.2274, "fy"=357.2274, "model"=4}, {"ID"=41, "Profile"=521316504, "fps"=30, "RS Stream"=0, "RS Format"=0, "index"=1, "width"=480, "height"=270, "ppx"=237.96481, "ppy"=139.0124, "fx"=357.2274, "fy"=357.2274, "model"=4}, {"ID"=41, "Profile"=521325464, "fps"=30, "RS Stream"=0, "RS Format"=0, "index"=0, "width"=480, "height"=270, "ppx"=237.96481, "ppy"=139.0124, "fx"=357.2274, "fy"=357.2274, "model"=4}, {"ID"=41, "Profile"=521325976, "fps"=30, "RS Stream"=0, "RS Format"=0, "index"=0, "width"=480, "height"=270, "ppx"=237.96481, "ppy"=139.0124, "fx"=357.2274, "fy"=357.2274, "model"=4}, {"ID"=41, "Profile"=521338520, "fps"=30, "RS Stream"=0, "RS Format"=0, "index"=0, "width"=480, "height"=270, "ppx"=237.96481, "ppy"=139.0124, "fx"=357.2274, "fy"=357.2274, "model"=4}, {"ID"=41, "Profile"=521332632, "fps"=30, "RS Stream"=0, "RS Format"=0, "index"=0, "width"=480, "height"=270, "ppx"=237.96481, "ppy"=139.0124, "fx"=357.2274, "fy"=357.2274, "model"=4}, {"ID"=41, "Profile"=521330328, "fps"=15, "RS Stream"=0, "RS Format"=0, "index"=0, "width"=480, "height"=270, "ppx"=237.96481, "ppy"=139.0124, "fx"=357.2274, "fy"=357.2274, "model"=4}, {"ID"=41, "Profile"=521328536, "fps"=15, "RS Stream"=0, "RS Format"=0, "index"=0, "width"=480, "height"=270, "ppx"=0.0, "ppy"=0.0, "fx"=0.0, "fy"=0.0, "model"=0}, {"ID"=41, "Profile"=521318808, "fps"=15, "RS Stream"=0, "RS Format"=0, "index"=1, "width"=480, "height"=270, "ppx"=237.96481, "ppy"=139.0124, "fx"=357.2274, "fy"=357.2274, "model"=4}, {"ID"=42, "Profile"=521610936, "fps"=15, "RS Stream"=0, "RS Format"=0, "index"=2, "width"=480, "height"=270, "ppx"=237.96481, "ppy"=139.0124, "fx"=357.2274, "fy"=357.2274, "model"=4}, {"ID"=41, "Profile"=521324440, "fps"=15, "RS Stream"=0, "RS Format"=0, "index"=0, "width"=480, "height"=270, "ppx"=237.96481, "ppy"=139.0124, "fx"=357.2274, "fy"=357.2274, "model"=4}, {"ID"=41, "Profile"=521328792, "fps"=15, "RS Stream"=0, "RS Format"=0, "index"=0, "width"=480, "height"=270, "ppx"=237.96481, "ppy"=139.0124, "fx"=357.2274, "fy"=357.2274, "model"=4}, {"ID"=41, "Profile"=521324184, "fps"=15, "RS Stream"=0, "RS Format"=0, "index"=0, "width"=480, "height"=270, "ppx"=237.96481, "ppy"=139.0124, "fx"=357.2274, "fy"=357.2274, "model"=4}, {"ID"=41, "Profile"=521323672, "fps"=15, "RS Stream"=0, "RS Format"=0, "index"=0, "width"=480, "height"=270, "ppx"=237.96481, "ppy"=139.0124, "fx"=357.2274, "fy"=357.2274, "model"=4}, {"ID"=41, "Profile"=521331352, "fps"=6, "RS Stream"=0, "RS Format"=0, "index"=0, "width"=480, "height"=270, "ppx"=237.96481, "ppy"=139.0124, "fx"=357.2274, "fy"=357.2274, "model"=4}, {"ID"=41, "Profile"=521324696, "fps"=6, "RS Stream"=0, "RS Format"=0, "index"=0, "width"=480, "height"=270, "ppx"=0.0, "ppy"=0.0, "fx"=0.0, "fy"=0.0, "model"=0}, {"ID"=42, "Profile"=521602488, "fps"=6, "RS Stream"=0, "RS Format"=0, "index"=2, "width"=480, "height"=270, "ppx"=237.96481, "ppy"=139.0124, "fx"=357.2274, "fy"=357.2274, "model"=4}, {"ID"=41, "Profile"=521314968, "fps"=6, "RS Stream"=0, "RS Format"=0, "index"=1, "width"=480, "height"=270, "ppx"=237.96481, "ppy"=139.0124, "fx"=357.2274, "fy"=357.2274, "model"=4}, {"ID"=41, "Profile"=521330072, "fps"=6, "RS Stream"=0, "RS Format"=0, "index"=0, "width"=480, "height"=270, "ppx"=237.96481, "ppy"=139.0124, "fx"=357.2274, "fy"=357.2274, "model"=4}, {"ID"=41, "Profile"=521326488, "fps"=6, "RS Stream"=0, "RS Format"=0, "index"=0, "width"=480, "height"=270, "ppx"=237.96481, "ppy"=139.0124, "fx"=357.2274, "fy"=357.2274, "model"=4}, {"ID"=41, "Profile"=521329304, "fps"=6, "RS Stream"=0, "RS Format"=0, "index"=0, "width"=480, "height"=270, "ppx"=237.96481, "ppy"=139.0124, "fx"=357.2274, "fy"=357.2274, "model"=4}, {"ID"=41, "Profile"=521329048, "fps"=6, "RS Stream"=0, "RS Format"=0, "index"=0, "width"=480, "height"=270, "ppx"=237.96481, "ppy"=139.0124, "fx"=357.2274, "fy"=357.2274, "model"=4}, {"ID"=41, "Profile"=521307032, "fps"=90, "RS Stream"=0, "RS Format"=0, "index"=0, "width"=424, "height"=240, "ppx"=210.19093, "ppy"=123.56658, "fx"=317.53546, "fy"=317.53546, "model"=4}, {"ID"=41, "Profile"=521322136, "fps"=90, "RS Stream"=0, "RS Format"=0, "index"=0, "width"=424, "height"=240, "ppx"=0.0, "ppy"=0.0, "fx"=0.0, "fy"=0.0, "model"=0}, {"ID"=42, "Profile"=521601976, "fps"=90, "RS Stream"=0, "RS Format"=0, "index"=2, "width"=424, "height"=240, "ppx"=210.19093, "ppy"=123.56658, "fx"=317.53546, "fy"=317.53546, "model"=4}, {"ID"=41, "Profile"=521315736, "fps"=90, "RS Stream"=0, "RS Format"=0, "index"=1, "width"=424, "height"=240, "ppx"=210.19093, "ppy"=123.56658, "fx"=317.53546, "fy"=317.53546, "model"=4}, {"ID"=41, "Profile"=521338776, "fps"=90, "RS Stream"=0, "RS Format"=0, "index"=0, "width"=424, "height"=240, "ppx"=210.19093, "ppy"=123.56658, "fx"=317.53546, "fy"=317.53546, "model"=4}, {"ID"=41, "Profile"=521307288, "fps"=90, "RS Stream"=0, "RS Format"=0, "index"=0, "width"=424, "height"=240, "ppx"=210.19093, "ppy"=123.56658, "fx"=317.53546, "fy"=317.53546, "model"=4}, {"ID"=41, "Profile"=521307544, "fps"=90, "RS Stream"=0, "RS Format"=0, "index"=0, "width"=424, "height"=240, "ppx"=210.19093, "ppy"=123.56658, "fx"=317.53546, "fy"=317.53546, "model"=4}, {"ID"=41, "Profile"=521321624, "fps"=90, "RS Stream"=0, "RS Format"=0, "index"=0, "width"=424, "height"=240, "ppx"=210.19093, "ppy"=123.56658, "fx"=317.53546, "fy"=317.53546, "model"=4}, {"ID"=41, "Profile"=521323928, "fps"=60, "RS Stream"=0, "RS Format"=0, "index"=0, "width"=424, "height"=240, "ppx"=210.19093, "ppy"=123.56658, "fx"=317.53546, "fy"=317.53546, "model"=4}, {"ID"=41, "Profile"=521339032, "fps"=60, "RS Stream"=0, "RS Format"=0, "index"=0, "width"=424, "height"=240, "ppx"=0.0, "ppy"=0.0, "fx"=0.0, "fy"=0.0, "model"=0}, {"ID"=42, "Profile"=521614008, "fps"=60, "RS Stream"=0, "RS Format"=0, "index"=2, "width"=424, "height"=240, "ppx"=210.19093, "ppy"=123.56658, "fx"=317.53546, "fy"=317.53546, "model"=4}, {"ID"=41, "Profile"=521313688, "fps"=60, "RS Stream"=0, "RS Format"=0, "index"=1, "width"=424, "height"=240, "ppx"=210.19093, "ppy"=123.56658, "fx"=317.53546, "fy"=317.53546, "model"=4}, {"ID"=41, "Profile"=521335192, "fps"=60, "RS Stream"=0, "RS Format"=0, "index"=0, "width"=424, "height"=240, "ppx"=210.19093, "ppy"=123.56658, "fx"=317.53546, "fy"=317.53546, "model"=4}, {"ID"=41, "Profile"=521337240, "fps"=60, "RS Stream"=0, "RS Format"=0, "index"=0, "width"=424, "height"=240, "ppx"=210.19093, "ppy"=123.56658, "fx"=317.53546, "fy"=317.53546, "model"=4}, {"ID"=41, "Profile"=521334680, "fps"=60, "RS Stream"=0, "RS Format"=0, "index"=0, "width"=424, "height"=240, "ppx"=210.19093, "ppy"=123.56658, "fx"=317.53546, "fy"=317.53546, "model"=4}, {"ID"=41, "Profile"=521334936, "fps"=60, "RS Stream"=0, "RS Format"=0, "index"=0, "width"=424, "height"=240, "ppx"=210.19093, "ppy"=123.56658, "fx"=317.53546, "fy"=317.53546, "model"=4}, {"ID"=41, "Profile"=521324952, "fps"=30, "RS Stream"=0, "RS Format"=0, "index"=0, "width"=424, "height"=240, "ppx"=210.19093, "ppy"=123.56658, "fx"=317.53546, "fy"=317.53546, "model"=4}, {"ID"=41, "Profile"=521335448, "fps"=30, "RS Stream"=0, "RS Format"=0, "index"=0, "width"=424, "height"=240, "ppx"=0.0, "ppy"=0.0, "fx"=0.0, "fy"=0.0, "model"=0}, {"ID"=42, "Profile"=521614264, "fps"=30, "RS Stream"=0, "RS Format"=0, "index"=2, "width"=424, "height"=240, "ppx"=210.19093, "ppy"=123.56658, "fx"=317.53546, "fy"=317.53546, "model"=4}, {"ID"=41, "Profile"=521314712, "fps"=30, "RS Stream"=0, "RS Format"=0, "index"=1, "width"=424, "height"=240, "ppx"=210.19093, "ppy"=123.56658, "fx"=317.53546, "fy"=317.53546, "model"=4}, {"ID"=41, "Profile"=521335704, "fps"=30, "RS Stream"=0, "RS Format"=0, "index"=0, "width"=424, "height"=240, "ppx"=210.19093, "ppy"=123.56658, "fx"=317.53546, "fy"=317.53546, "model"=4}, {"ID"=41, "Profile"=521327000, "fps"=30, "RS Stream"=0, "RS Format"=0, "index"=0, "width"=424, "height"=240, "ppx"=210.19093, "ppy"=123.56658, "fx"=317.53546, "fy"=317.53546, "model"=4}, {"ID"=41, "Profile"=521333656, "fps"=30, "RS Stream"=0, "RS Format"=0, "index"=0, "width"=424, "height"=240, "ppx"=210.19093, "ppy"=123.56658, "fx"=317.53546, "fy"=317.53546, "model"=4}, {"ID"=41, "Profile"=521336216, "fps"=30, "RS Stream"=0, "RS Format"=0, "index"=0, "width"=424, "height"=240, "ppx"=210.19093, "ppy"=123.56658, "fx"=317.53546, "fy"=317.53546, "model"=4}, {"ID"=41, "Profile"=521332376, "fps"=15, "RS Stream"=0, "RS Format"=0, "index"=0, "width"=424, "height"=240, "ppx"=210.19093, "ppy"=123.56658, "fx"=317.53546, "fy"=317.53546, "model"=4}, {"ID"=41, "Profile"=521339288, "fps"=15, "RS Stream"=0, "RS Format"=0, "index"=0, "width"=424, "height"=240, "ppx"=0.0, "ppy"=0.0, "fx"=0.0, "fy"=0.0, "model"=0}, {"ID"=42, "Profile"=521611192, "fps"=15, "RS Stream"=0, "RS Format"=0, "index"=2, "width"=424, "height"=240, "ppx"=210.19093, "ppy"=123.56658, "fx"=317.53546, "fy"=317.53546, "model"=4}, {"ID"=41, "Profile"=521310104, "fps"=15, "RS Stream"=0, "RS Format"=0, "index"=1, "width"=424, "height"=240, "ppx"=210.19093, "ppy"=123.56658, "fx"=317.53546, "fy"=317.53546, "model"=4}, {"ID"=41, "Profile"=521325208, "fps"=15, "RS Stream"=0, "RS Format"=0, "index"=0, "width"=424, "height"=240, "ppx"=210.19093, "ppy"=123.56658, "fx"=317.53546, "fy"=317.53546, "model"=4}, {"ID"=41, "Profile"=521329560, "fps"=15, "RS Stream"=0, "RS Format"=0, "index"=0, "width"=424, "height"=240, "ppx"=210.19093, "ppy"=123.56658, "fx"=317.53546, "fy"=317.53546, "model"=4}, {"ID"=41, "Profile"=521338008, "fps"=15, "RS Stream"=0, "RS Format"=0, "index"=0, "width"=424, "height"=240, "ppx"=210.19093, "ppy"=123.56658, "fx"=317.53546, "fy"=317.53546, "model"=4}, {"ID"=41, "Profile"=521335960, "fps"=15, "RS Stream"=0, "RS Format"=0, "index"=0, "width"=424, "height"=240, "ppx"=210.19093, "ppy"=123.56658, "fx"=317.53546, "fy"=317.53546, "model"=4}, {"ID"=41, "Profile"=521333400, "fps"=6, "RS Stream"=0, "RS Format"=0, "index"=0, "width"=424, "height"=240, "ppx"=210.19093, "ppy"=123.56658, "fx"=317.53546, "fy"=317.53546, "model"=4}, {"ID"=41, "Profile"=521334168, "fps"=6, "RS Stream"=0, "RS Format"=0, "index"=0, "width"=424, "height"=240, "ppx"=0.0, "ppy"=0.0, "fx"=0.0, "fy"=0.0, "model"=0}, {"ID"=42, "Profile"=521602232, "fps"=6, "RS Stream"=0, "RS Format"=0, "index"=2, "width"=424, "height"=240, "ppx"=210.19093, "ppy"=123.56658, "fx"=317.53546, "fy"=317.53546, "model"=4}, {"ID"=41, "Profile"=521311384, "fps"=6, "RS Stream"=0, "RS Format"=0, "index"=1, "width"=424, "height"=240, "ppx"=210.19093, "ppy"=123.56658, "fx"=317.53546, "fy"=317.53546, "model"=4}, {"ID"=41, "Profile"=521334424, "fps"=6, "RS Stream"=0, "RS Format"=0, "index"=0, "width"=424, "height"=240, "ppx"=210.19093, "ppy"=123.56658, "fx"=317.53546, "fy"=317.53546, "model"=4}, {"ID"=41, "Profile"=521323160, "fps"=6, "RS Stream"=0, "RS Format"=0, "index"=0, "width"=424, "height"=240, "ppx"=210.19093, "ppy"=123.56658, "fx"=317.53546, "fy"=317.53546, "model"=4}, {"ID"=41, "Profile"=521327512, "fps"=6, "RS Stream"=0, "RS Format"=0, "index"=0, "width"=424, "height"=240, "ppx"=210.19093, "ppy"=123.56658, "fx"=317.53546, "fy"=317.53546, "model"=4}, {"ID"=41, "Profile"=521327256, "fps"=6, "RS Stream"=0, "RS Format"=0, "index"=0, "width"=424, "height"=240, "ppx"=210.19093, "ppy"=123.56658, "fx"=317.53546, "fy"=317.53546, "model"=4}, {"ID"=40, "Profile"=521312408, "fps"=30, "RS Stream"=0, "RS Format"=0, "index"=0, "width"=1280, "height"=720, "ppx"=634.5728, "ppy"=370.69974, "fx"=952.6064, "fy"=952.6064, "model"=4}, {"ID"=40, "Profile"=521319832, "fps"=30, "RS Stream"=0, "RS Format"=0, "index"=0, "width"=1280, "height"=720, "ppx"=634.5728, "ppy"=370.69974, "fx"=952.6064, "fy"=952.6064, "model"=4}, {"ID"=40, "Profile"=521309336, "fps"=15, "RS Stream"=0, "RS Format"=0, "index"=0, "width"=1280, "height"=720, "ppx"=634.5728, "ppy"=370.69974, "fx"=952.6064, "fy"=952.6064, "model"=4}, {"ID"=40, "Profile"=521316248, "fps"=15, "RS Stream"=0, "RS Format"=0, "index"=0, "width"=1280, "height"=720, "ppx"=634.5728, "ppy"=370.69974, "fx"=952.6064, "fy"=952.6064, "model"=4}, {"ID"=40, "Profile"=521309080, "fps"=6, "RS Stream"=0, "RS Format"=0, "index"=0, "width"=1280, "height"=720, "ppx"=634.5728, "ppy"=370.69974, "fx"=952.6064, "fy"=952.6064, "model"=4}, {"ID"=40, "Profile"=521315224, "fps"=6, "RS Stream"=0, "RS Format"=0, "index"=0, "width"=1280, "height"=720, "ppx"=634.5728, "ppy"=370.69974, "fx"=952.6064, "fy"=952.6064, "model"=4}, {"ID"=40, "Profile"=521317784, "fps"=90, "RS Stream"=0, "RS Format"=0, "index"=0, "width"=848, "height"=480, "ppx"=420.38187, "ppy"=247.13316, "fx"=635.0709, "fy"=635.0709, "model"=4}, {"ID"=40, "Profile"=521322392, "fps"=90, "RS Stream"=0, "RS Format"=0, "index"=0, "width"=848, "height"=480, "ppx"=420.38187, "ppy"=247.13316, "fx"=635.0709, "fy"=635.0709, "model"=4}, {"ID"=40, "Profile"=521321880, "fps"=60, "RS Stream"=0, "RS Format"=0, "index"=0, "width"=848, "height"=480, "ppx"=420.38187, "ppy"=247.13316, "fx"=635.0709, "fy"=635.0709, "model"=4}, {"ID"=40, "Profile"=521318040, "fps"=60, "RS Stream"=0, "RS Format"=0, "index"=0, "width"=848, "height"=480, "ppx"=420.38187, "ppy"=247.13316, "fx"=635.0709, "fy"=635.0709, "model"=4}, {"ID"=40, "Profile"=521312920, "fps"=30, "RS Stream"=0, "RS Format"=0, "index"=0, "width"=848, "height"=480, "ppx"=420.38187, "ppy"=247.13316, "fx"=635.0709, "fy"=635.0709, "model"=4}, {"ID"=40, "Profile"=521320856, "fps"=30, "RS Stream"=0, "RS Format"=0, "index"=0, "width"=848, "height"=480, "ppx"=420.38187, "ppy"=247.13316, "fx"=635.0709, "fy"=635.0709, "model"=4}, {"ID"=40, "Profile"=521319576, "fps"=15, "RS Stream"=0, "RS Format"=0, "index"=0, "width"=848, "height"=480, "ppx"=420.38187, "ppy"=247.13316, "fx"=635.0709, "fy"=635.0709, "model"=4}, {"ID"=40, "Profile"=521308056, "fps"=15, "RS Stream"=0, "RS Format"=0, "index"=0, "width"=848, "height"=480, "ppx"=420.38187, "ppy"=247.13316, "fx"=635.0709, "fy"=635.0709, "model"=4}, {"ID"=40, "Profile"=521312664, "fps"=6, "RS Stream"=0, "RS Format"=0, "index"=0, "width"=848, "height"=480, "ppx"=420.38187, "ppy"=247.13316, "fx"=635.0709, "fy"=635.0709, "model"=4}, {"ID"=40, "Profile"=521308824, "fps"=6, "RS Stream"=0, "RS Format"=0, "index"=0, "width"=848, "height"=480, "ppx"=420.38187, "ppy"=247.13316, "fx"=635.0709, "fy"=635.0709, "model"=4}, {"ID"=40, "Profile"=521308568, "fps"=90, "RS Stream"=0, "RS Format"=0, "index"=0, "width"=640, "height"=480, "ppx"=316.38187, "ppy"=247.13316, "fx"=635.0709, "fy"=635.0709, "model"=4}, {"ID"=40, "Profile"=521313432, "fps"=90, "RS Stream"=0, "RS Format"=0, "index"=0, "width"=640, "height"=480, "ppx"=316.38187, "ppy"=247.13316, "fx"=635.0709, "fy"=635.0709, "model"=4}, {"ID"=40, "Profile"=521315480, "fps"=60, "RS Stream"=0, "RS Format"=0, "index"=0, "width"=640, "height"=480, "ppx"=316.38187, "ppy"=247.13316, "fx"=635.0709, "fy"=635.0709, "model"=4}, {"ID"=40, "Profile"=521318552, "fps"=60, "RS Stream"=0, "RS Format"=0, "index"=0, "width"=640, "height"=480, "ppx"=316.38187, "ppy"=247.13316, "fx"=635.0709, "fy"=635.0709, "model"=4}, {"ID"=40, "Profile"=521311128, "fps"=30, "RS Stream"=0, "RS Format"=0, "index"=0, "width"=640, "height"=480, "ppx"=316.38187, "ppy"=247.13316, "fx"=635.0709, "fy"=635.0709, "model"=4}, {"ID"=40, "Profile"=521309848, "fps"=30, "RS Stream"=0, "RS Format"=0, "index"=0, "width"=640, "height"=480, "ppx"=316.38187, "ppy"=247.13316, "fx"=635.0709, "fy"=635.0709, "model"=4}, {"ID"=40, "Profile"=521317528, "fps"=15, "RS Stream"=0, "RS Format"=0, "index"=0, "width"=640, "height"=480, "ppx"=316.38187, "ppy"=247.13316, "fx"=635.0709, "fy"=635.0709, "model"=4}, {"ID"=40, "Profile"=521316760, "fps"=15, "RS Stream"=0, "RS Format"=0, "index"=0, "width"=640, "height"=480, "ppx"=316.38187, "ppy"=247.13316, "fx"=635.0709, "fy"=635.0709, "model"=4}, {"ID"=40, "Profile"=521311896, "fps"=6, "RS Stream"=0, "RS Format"=0, "index"=0, "width"=640, "height"=480, "ppx"=316.38187, "ppy"=247.13316, "fx"=635.0709, "fy"=635.0709, "model"=4}, {"ID"=40, "Profile"=521307800, "fps"=6, "RS Stream"=0, "RS Format"=0, "index"=0, "width"=640, "height"=480, "ppx"=316.38187, "ppy"=247.13316, "fx"=635.0709, "fy"=635.0709, "model"=4}, {"ID"=40, "Profile"=521290648, "fps"=90, "RS Stream"=0, "RS Format"=0, "index"=0, "width"=640, "height"=360, "ppx"=317.2864, "ppy"=185.34987, "fx"=476.3032, "fy"=476.3032, "model"=4}, {"ID"=40, "Profile"=521306520, "fps"=90, "RS Stream"=0, "RS Format"=0, "index"=0, "width"=640, "height"=360, "ppx"=317.2864, "ppy"=185.34987, "fx"=476.3032, "fy"=476.3032, "model"=4}, {"ID"=40, "Profile"=521293208, "fps"=60, "RS Stream"=0, "RS Format"=0, "index"=0, "width"=640, "height"=360, "ppx"=317.2864, "ppy"=185.34987, "fx"=476.3032, "fy"=476.3032, "model"=4}, {"ID"=40, "Profile"=521292952, "fps"=60, "RS Stream"=0, "RS Format"=0, "index"=0, "width"=640, "height"=360, "ppx"=317.2864, "ppy"=185.34987, "fx"=476.3032, "fy"=476.3032, "model"=4}, {"ID"=40, "Profile"=521294232, "fps"=30, "RS Stream"=0, "RS Format"=0, "index"=0, "width"=640, "height"=360, "ppx"=317.2864, "ppy"=185.34987, "fx"=476.3032, "fy"=476.3032, "model"=4}, {"ID"=40, "Profile"=521293720, "fps"=30, "RS Stream"=0, "RS Format"=0, "index"=0, "width"=640, "height"=360, "ppx"=317.2864, "ppy"=185.34987, "fx"=476.3032, "fy"=476.3032, "model"=4}, {"ID"=40, "Profile"=521317016, "fps"=15, "RS Stream"=0, "RS Format"=0, "index"=0, "width"=640, "height"=360, "ppx"=317.2864, "ppy"=185.34987, "fx"=476.3032, "fy"=476.3032, "model"=4}, {"ID"=40, "Profile"=521308312, "fps"=15, "RS Stream"=0, "RS Format"=0, "index"=0, "width"=640, "height"=360, "ppx"=317.2864, "ppy"=185.34987, "fx"=476.3032, "fy"=476.3032, "model"=4}, {"ID"=40, "Profile"=521311640, "fps"=6, "RS Stream"=0, "RS Format"=0, "index"=0, "width"=640, "height"=360, "ppx"=317.2864, "ppy"=185.34987, "fx"=476.3032, "fy"=476.3032, "model"=4}, {"ID"=40, "Profile"=521313944, "fps"=6, "RS Stream"=0, "RS Format"=0, "index"=0, "width"=640, "height"=360, "ppx"=317.2864, "ppy"=185.34987, "fx"=476.3032, "fy"=476.3032, "model"=4}, {"ID"=40, "Profile"=521293464, "fps"=90, "RS Stream"=0, "RS Format"=0, "index"=0, "width"=480, "height"=270, "ppx"=237.96481, "ppy"=139.0124, "fx"=357.2274, "fy"=357.2274, "model"=4}, {"ID"=40, "Profile"=521297560, "fps"=90, "RS Stream"=0, "RS Format"=0, "index"=0, "width"=480, "height"=270, "ppx"=237.96481, "ppy"=139.0124, "fx"=357.2274, "fy"=357.2274, "model"=4}, {"ID"=40, "Profile"=521302680, "fps"=60, "RS Stream"=0, "RS Format"=0, "index"=0, "width"=480, "height"=270, "ppx"=237.96481, "ppy"=139.0124, "fx"=357.2274, "fy"=357.2274, "model"=4}, {"ID"=40, "Profile"=521300376, "fps"=60, "RS Stream"=0, "RS Format"=0, "index"=0, "width"=480, "height"=270, "ppx"=237.96481, "ppy"=139.0124, "fx"=357.2274, "fy"=357.2274, "model"=4}, {"ID"=40, "Profile"=521302936, "fps"=30, "RS Stream"=0, "RS Format"=0, "index"=0, "width"=480, "height"=270, "ppx"=237.96481, "ppy"=139.0124, "fx"=357.2274, "fy"=357.2274, "model"=4}, {"ID"=40, "Profile"=521301144, "fps"=30, "RS Stream"=0, "RS Format"=0, "index"=0, "width"=480, "height"=270, "ppx"=237.96481, "ppy"=139.0124, "fx"=357.2274, "fy"=357.2274, "model"=4}, {"ID"=40, "Profile"=521303192, "fps"=15, "RS Stream"=0, "RS Format"=0, "index"=0, "width"=480, "height"=270, "ppx"=237.96481, "ppy"=139.0124, "fx"=357.2274, "fy"=357.2274, "model"=4}, {"ID"=40, "Profile"=521304984, "fps"=15, "RS Stream"=0, "RS Format"=0, "index"=0, "width"=480, "height"=270, "ppx"=237.96481, "ppy"=139.0124, "fx"=357.2274, "fy"=357.2274, "model"=4}, {"ID"=40, "Profile"=521304216, "fps"=6, "RS Stream"=0, "RS Format"=0, "index"=0, "width"=480, "height"=270, "ppx"=237.96481, "ppy"=139.0124, "fx"=357.2274, "fy"=357.2274, "model"=4}, {"ID"=40, "Profile"=521303704, "fps"=6, "RS Stream"=0, "RS Format"=0, "index"=0, "width"=480, "height"=270, "ppx"=237.96481, "ppy"=139.0124, "fx"=357.2274, "fy"=357.2274, "model"=4}, {"ID"=40, "Profile"=521306264, "fps"=90, "RS Stream"=0, "RS Format"=0, "index"=0, "width"=424, "height"=240, "ppx"=210.19093, "ppy"=123.56658, "fx"=317.53546, "fy"=317.53546, "model"=4}, {"ID"=40, "Profile"=521301912, "fps"=90, "RS Stream"=0, "RS Format"=0, "index"=0, "width"=424, "height"=240, "ppx"=210.19093, "ppy"=123.56658, "fx"=317.53546, "fy"=317.53546, "model"=4}, {"ID"=40, "Profile"=521292184, "fps"=60, "RS Stream"=0, "RS Format"=0, "index"=0, "width"=424, "height"=240, "ppx"=210.19093, "ppy"=123.56658, "fx"=317.53546, "fy"=317.53546, "model"=4}, {"ID"=40, "Profile"=521291928, "fps"=60, "RS Stream"=0, "RS Format"=0, "index"=0, "width"=424, "height"=240, "ppx"=210.19093, "ppy"=123.56658, "fx"=317.53546, "fy"=317.53546, "model"=4}, {"ID"=40, "Profile"=521296792, "fps"=30, "RS Stream"=0, "RS Format"=0, "index"=0, "width"=424, "height"=240, "ppx"=210.19093, "ppy"=123.56658, "fx"=317.53546, "fy"=317.53546, "model"=4}, {"ID"=40, "Profile"=521300120, "fps"=30, "RS Stream"=0, "RS Format"=0, "index"=0, "width"=424, "height"=240, "ppx"=210.19093, "ppy"=123.56658, "fx"=317.53546, "fy"=317.53546, "model"=4}, {"ID"=40, "Profile"=521300632, "fps"=15, "RS Stream"=0, "RS Format"=0, "index"=0, "width"=424, "height"=240, "ppx"=210.19093, "ppy"=123.56658, "fx"=317.53546, "fy"=317.53546, "model"=4}, {"ID"=40, "Profile"=521302424, "fps"=15, "RS Stream"=0, "RS Format"=0, "index"=0, "width"=424, "height"=240, "ppx"=210.19093, "ppy"=123.56658, "fx"=317.53546, "fy"=317.53546, "model"=4}, {"ID"=40, "Profile"=521300888, "fps"=6, "RS Stream"=0, "RS Format"=0, "index"=0, "width"=424, "height"=240, "ppx"=210.19093, "ppy"=123.56658, "fx"=317.53546, "fy"=317.53546, "model"=4}, {"ID"=40, "Profile"=521292696, "fps"=6, "RS Stream"=0, "RS Format"=0, "index"=0, "width"=424, "height"=240, "ppx"=210.19093, "ppy"=123.56658, "fx"=317.53546, "fy"=317.53546, "model"=4}] {"model" items=["RS_DISTORTION_NONE", "RS_DISTORTION_MODIFIED_BROWN_CONRADY", "RS_DISTORTION_INVERSE_BROWN_CONRADY", "RS_DISTORTION_FTHETA", "RS_DISTORTION_BROWN_CONRADY", "RS_DISTORTION_COUNT"]; "RS Stream" items=["    RS2_STREAM_ANY,", "    RS2_STREAM_DEPTH                            , /**< Native stream of depth data produced by RealSense device */", "    RS2_STREAM_COLOR                            , /**< Native stream of color data captured by RealSense device */", "    RS2_STREAM_INFRARED                         , /**< Native stream of infrared data captured by RealSense device */", "    RS2_STREAM_FISHEYE                          , /**< Native stream of fish-eye (wide) data captured from the dedicate motion camera */", "    RS2_STREAM_GYRO                             , /**< Native stream of gyroscope motion data produced by RealSense device */", "    RS2_STREAM_ACCEL                            , /**< Native stream of accelerometer motion data produced by RealSense device */", "    RS2_STREAM_GPIO                             , /**< Signals from external device connected through GPIO */", "    RS2_STREAM_POSE                             , /**< 6 Degrees of Freedom pose data, calculated by RealSense device */", "    RS2_STREAM_CONFIDENCE,", "    RS2_STREAM_COUNT"]}) -> (1 "RGB ext.":T1(array[cluster])=[{"width"=424, "height"=240, "fps"=6, "Profile"=521292696, "ppx"=210.19093, "ppy"=123.56658, "fx"=317.53546, "fy"=317.53546, "model"=4}, {"width"=424, "height"=240, "fps"=15, "Profile"=521302424, "ppx"=210.19093, "ppy"=123.56658, "fx"=317.53546, "fy"=317.53546, "model"=4}, {"width"=424, "height"=240, "fps"=30, "Profile"=521300120, "ppx"=210.19093, "ppy"=123.56658, "fx"=317.53546, "fy"=317.53546, "model"=4}, {"width"=424, "height"=240, "fps"=60, "Profile"=521291928, "ppx"=210.19093, "ppy"=123.56658, "fx"=317.53546, "fy"=317.53546, "model"=4}, {"width"=424, "height"=240, "fps"=90, "Profile"=521301912, "ppx"=210.19093, "ppy"=123.56658, "fx"=317.53546, "fy"=317.53546, "model"=4}, {"width"=480, "height"=270, "fps"=6, "Profile"=521303704, "ppx"=237.96481, "ppy"=139.0124, "fx"=357.2274, "fy"=357.2274, "model"=4}, {"width"=480, "height"=270, "fps"=15, "Profile"=521304984, "ppx"=237.96481, "ppy"=139.0124, "fx"=357.2274, "fy"=357.2274, "model"=4}, {"width"=480, "height"=270, "fps"=30, "Profile"=521301144, "ppx"=237.96481, "ppy"=139.0124, "fx"=357.2274, "fy"=357.2274, "model"=4}, {"width"=480, "height"=270, "fps"=60, "Profile"=521300376, "ppx"=237.96481, "ppy"=139.0124, "fx"=357.2274, "fy"=357.2274, "model"=4}, {"width"=480, "height"=270, "fps"=90, "Profile"=521297560, "ppx"=237.96481, "ppy"=139.0124, "fx"=357.2274, "fy"=357.2274, "model"=4}, {"width"=640, "height"=360, "fps"=6, "Profile"=521313944, "ppx"=317.2864, "ppy"=185.34987, "fx"=476.3032, "fy"=476.3032, "model"=4}, {"width"=640, "height"=360, "fps"=15, "Profile"=521308312, "ppx"=317.2864, "ppy"=185.34987, "fx"=476.3032, "fy"=476.3032, "model"=4}, {"width"=640, "height"=360, "fps"=30, "Profile"=521293720, "ppx"=317.2864, "ppy"=185.34987, "fx"=476.3032, "fy"=476.3032, "model"=4}, {"width"=640, "height"=360, "fps"=60, "Profile"=521292952, "ppx"=317.2864, "ppy"=185.34987, "fx"=476.3032, "fy"=476.3032, "model"=4}, {"width"=640, "height"=360, "fps"=90, "Profile"=521306520, "ppx"=317.2864, "ppy"=185.34987, "fx"=476.3032, "fy"=476.3032, "model"=4}, {"width"=640, "height"=480, "fps"=6, "Profile"=521307800, "ppx"=316.38187, "ppy"=247.13316, "fx"=635.0709, "fy"=635.0709, "model"=4}, {"width"=640, "height"=480, "fps"=15, "Profile"=521316760, "ppx"=316.38187, "ppy"=247.13316, "fx"=635.0709, "fy"=635.0709, "model"=4}, {"width"=640, "height"=480, "fps"=30, "Profile"=521309848, "ppx"=316.38187, "ppy"=247.13316, "fx"=635.0709, "fy"=635.0709, "model"=4}, {"width"=640, "height"=480, "fps"=60, "Profile"=521318552, "ppx"=316.38187, "ppy"=247.13316, "fx"=635.0709, "fy"=635.0709, "model"=4}, {"width"=640, "height"=480, "fps"=90, "Profile"=521313432, "ppx"=316.38187, "ppy"=247.13316, "fx"=635.0709, "fy"=635.0709, "model"=4}, {"width"=848, "height"=480, "fps"=6, "Profile"=521308824, "ppx"=420.38187, "ppy"=247.13316, "fx"=635.0709, "fy"=635.0709, "model"=4}, {"width"=848, "height"=480, "fps"=15, "Profile"=521308056, "ppx"=420.38187, "ppy"=247.13316, "fx"=635.0709, "fy"=635.0709, "model"=4}, {"width"=848, "height"=480, "fps"=30, "Profile"=521320856, "ppx"=420.38187, "ppy"=247.13316, "fx"=635.0709, "fy"=635.0709, "model"=4}, {"width"=848, "height"=480, "fps"=60, "Profile"=521318040, "ppx"=420.38187, "ppy"=247.13316, "fx"=635.0709, "fy"=635.0709, "model"=4}, {"width"=848, "height"=480, "fps"=90, "Profile"=521322392, "ppx"=420.38187, "ppy"=247.13316, "fx"=635.0709, "fy"=635.0709, "model"=4}, {"width"=1280, "height"=720, "fps"=6, "Profile"=521315224, "ppx"=634.5728, "ppy"=370.69974, "fx"=952.6064, "fy"=952.6064, "model"=4}, {"width"=1280, "height"=720, "fps"=15, "Profile"=521316248, "ppx"=634.5728, "ppy"=370.69974, "fx"=952.6064, "fy"=952.6064, "model"=4}, {"width"=1280, "height"=720, "fps"=30, "Profile"=521319832, "ppx"=634.5728, "ppy"=370.69974, "fx"=952.6064, "fy"=952.6064, "model"=4}], 3 "RGB ext.":string[](array[string])=["424 x 240 @6fps", "424 x 240 @15fps", "424 x 240 @30fps", "424 x 240 @60fps", "424 x 240 @90fps", "480 x 270 @6fps", "480 x 270 @15fps", "480 x 270 @30fps", "480 x 270 @60fps", "480 x 270 @90fps", "640 x 360 @6fps", "640 x 360 @15fps", "640 x 360 @30fps", "640 x 360 @60fps", "640 x 360 @90fps", "640 x 480 @6fps", "640 x 480 @15fps", "640 x 480 @30fps", "640 x 480 @60fps", "640 x 480 @90fps", "848 x 480 @6fps", "848 x 480 @15fps", "848 x 480 @30fps", "848 x 480 @60fps", "848 x 480 @90fps", "1280 x 720 @6fps", "1280 x 720 @15fps", "1280 x 720 @30fps"], 4 "Unrectified L IR":T1(array[cluster])=[{"width"=424, "height"=240, "fps"=6, "Profile"=521292696, "ppx"=210.19093, "ppy"=123.56658, "fx"=317.53546, "fy"=317.53546, "model"=4}, {"width"=424, "height"=240, "fps"=15, "Profile"=521302424, "ppx"=210.19093, "ppy"=123.56658, "fx"=317.53546, "fy"=317.53546, "model"=4}, {"width"=424, "height"=240, "fps"=30, "Profile"=521300120, "ppx"=210.19093, "ppy"=123.56658, "fx"=317.53546, "fy"=317.53546, "model"=4}, {"width"=424, "height"=240, "fps"=60, "Profile"=521291928, "ppx"=210.19093, "ppy"=123.56658, "fx"=317.53546, "fy"=317.53546, "model"=4}, {"width"=424, "height"=240, "fps"=90, "Profile"=521301912, "ppx"=210.19093, "ppy"=123.56658, "fx"=317.53546, "fy"=317.53546, "model"=4}, {"width"=480, "height"=270, "fps"=6, "Profile"=521303704, "ppx"=237.96481, "ppy"=139.0124, "fx"=357.2274, "fy"=357.2274, "model"=4}, {"width"=480, "height"=270, "fps"=15, "Profile"=521304984, "ppx"=237.96481, "ppy"=139.0124, "fx"=357.2274, "fy"=357.2274, "model"=4}, {"width"=480, "height"=270, "fps"=30, "Profile"=521301144, "ppx"=237.96481, "ppy"=139.0124, "fx"=357.2274, "fy"=357.2274, "model"=4}, {"width"=480, "height"=270, "fps"=60, "Profile"=521300376, "ppx"=237.96481, "ppy"=139.0124, "fx"=357.2274, "fy"=357.2274, "model"=4}, {"width"=480, "height"=270, "fps"=90, "Profile"=521297560, "ppx"=237.96481, "ppy"=139.0124, "fx"=357.2274, "fy"=357.2274, "model"=4}, {"width"=640, "height"=360, "fps"=6, "Profile"=521313944, "ppx"=317.2864, "ppy"=185.34987, "fx"=476.3032, "fy"=476.3032, "model"=4}, {"width"=640, "height"=360, "fps"=15, "Profile"=521308312, "ppx"=317.2864, "ppy"=185.34987, "fx"=476.3032, "fy"=476.3032, "model"=4}, {"width"=640, "height"=360, "fps"=30, "Profile"=521293720, "ppx"=317.2864, "ppy"=185.34987, "fx"=476.3032, "fy"=476.3032, "model"=4}, {"width"=640, "height"=360, "fps"=60, "Profile"=521292952, "ppx"=317.2864, "ppy"=185.34987, "fx"=476.3032, "fy"=476.3032, "model"=4}, {"width"=640, "height"=360, "fps"=90, "Profile"=521306520, "ppx"=317.2864, "ppy"=185.34987, "fx"=476.3032, "fy"=476.3032, "model"=4}, {"width"=640, "height"=480, "fps"=6, "Profile"=521307800, "ppx"=316.38187, "ppy"=247.13316, "fx"=635.0709, "fy"=635.0709, "model"=4}, {"width"=640, "height"=480, "fps"=15, "Profile"=521316760, "ppx"=316.38187, "ppy"=247.13316, "fx"=635.0709, "fy"=635.0709, "model"=4}, {"width"=640, "height"=480, "fps"=30, "Profile"=521309848, "ppx"=316.38187, "ppy"=247.13316, "fx"=635.0709, "fy"=635.0709, "model"=4}, {"width"=640, "height"=480, "fps"=60, "Profile"=521318552, "ppx"=316.38187, "ppy"=247.13316, "fx"=635.0709, "fy"=635.0709, "model"=4}, {"width"=640, "height"=480, "fps"=90, "Profile"=521313432, "ppx"=316.38187, "ppy"=247.13316, "fx"=635.0709, "fy"=635.0709, "model"=4}, {"width"=848, "height"=480, "fps"=6, "Profile"=521308824, "ppx"=420.38187, "ppy"=247.13316, "fx"=635.0709, "fy"=635.0709, "model"=4}, {"width"=848, "height"=480, "fps"=15, "Profile"=521308056, "ppx"=420.38187, "ppy"=247.13316, "fx"=635.0709, "fy"=635.0709, "model"=4}, {"width"=848, "height"=480, "fps"=30, "Profile"=521320856, "ppx"=420.38187, "ppy"=247.13316, "fx"=635.0709, "fy"=635.0709, "model"=4}, {"width"=848, "height"=480, "fps"=60, "Profile"=521318040, "ppx"=420.38187, "ppy"=247.13316, "fx"=635.0709, "fy"=635.0709, "model"=4}, {"width"=848, "height"=480, "fps"=90, "Profile"=521322392, "ppx"=420.38187, "ppy"=247.13316, "fx"=635.0709, "fy"=635.0709, "model"=4}, {"width"=1280, "height"=720, "fps"=6, "Profile"=521315224, "ppx"=634.5728, "ppy"=370.69974, "fx"=952.6064, "fy"=952.6064, "model"=4}, {"width"=1280, "height"=720, "fps"=15, "Profile"=521316248, "ppx"=634.5728, "ppy"=370.69974, "fx"=952.6064, "fy"=952.6064, "model"=4}, {"width"=1280, "height"=720, "fps"=30, "Profile"=521319832, "ppx"=634.5728, "ppy"=370.69974, "fx"=952.6064, "fy"=952.6064, "model"=4}], 5 "Unrectified L IR":string[](array[string])=["424 x 240 @6fps", "424 x 240 @15fps", "424 x 240 @30fps", "424 x 240 @60fps", "424 x 240 @90fps", "480 x 270 @6fps", "480 x 270 @15fps", "480 x 270 @30fps", "480 x 270 @60fps", "480 x 270 @90fps", "640 x 360 @6fps", "640 x 360 @15fps", "640 x 360 @30fps", "640 x 360 @60fps", "640 x 360 @90fps", "640 x 480 @6fps", "640 x 480 @15fps", "640 x 480 @30fps", "640 x 480 @60fps", "640 x 480 @90fps", "848 x 480 @6fps", "848 x 480 @15fps", "848 x 480 @30fps", "848 x 480 @60fps", "848 x 480 @90fps", "1280 x 720 @6fps", "1280 x 720 @15fps", "1280 x 720 @30fps"], 6 "IR Left Array":string[](array[string])=["424 x 240 @6fps", "424 x 240 @15fps", "424 x 240 @30fps", "424 x 240 @60fps", "424 x 240 @90fps", "480 x 270 @6fps", "480 x 270 @15fps", "480 x 270 @30fps", "480 x 270 @60fps", "480 x 270 @90fps", "640 x 360 @6fps", "640 x 360 @15fps", "640 x 360 @30fps", "640 x 360 @60fps", "640 x 360 @90fps", "640 x 480 @6fps", "640 x 480 @15fps", "640 x 480 @30fps", "640 x 480 @60fps", "640 x 480 @90fps", "848 x 480 @6fps", "848 x 480 @15fps", "848 x 480 @30fps", "848 x 480 @60fps", "848 x 480 @90fps", "1280 x 720 @6fps", "1280 x 720 @15fps", "1280 x 720 @30fps", "1920 x 1080 @15fps", "1920 x 1080 @25fps"], 7 "IR Right Array":string[](array[string])=["424 x 240 @6fps", "424 x 240 @15fps", "424 x 240 @30fps", "424 x 240 @60fps", "424 x 240 @90fps", "480 x 270 @6fps", "480 x 270 @15fps", "480 x 270 @30fps", "480 x 270 @60fps", "480 x 270 @90fps", "640 x 360 @6fps", "640 x 360 @15fps", "640 x 360 @30fps", "640 x 360 @60fps", "640 x 360 @90fps", "640 x 480 @6fps", "640 x 480 @15fps", "640 x 480 @30fps", "640 x 480 @60fps", "640 x 480 @90fps", "848 x 480 @6fps", "848 x 480 @15fps", "848 x 480 @30fps", "848 x 480 @60fps", "848 x 480 @90fps", "1280 x 720 @6fps", "1280 x 720 @15fps", "1280 x 720 @30fps", "1920 x 1080 @15fps", "1920 x 1080 @25fps"], 10 "Unrectified R IR":string[](array[string])=["424 x 240 @6fps", "424 x 240 @15fps", "424 x 240 @30fps", "424 x 240 @60fps", "424 x 240 @90fps", "480 x 270 @6fps", "480 x 270 @15fps", "480 x 270 @30fps", "480 x 270 @60fps", "480 x 270 @90fps", "640 x 360 @6fps", "640 x 360 @15fps", "640 x 360 @30fps", "640 x 360 @60fps", "640 x 360 @90fps", "640 x 480 @6fps", "640 x 480 @15fps", "640 x 480 @30fps", "640 x 480 @60fps", "640 x 480 @90fps", "848 x 480 @6fps", "848 x 480 @15fps", "848 x 480 @30fps", "848 x 480 @60fps", "848 x 480 @90fps", "1280 x 720 @6fps", "1280 x 720 @15fps", "1280 x 720 @30fps"], 11 "Unrectified R  IR":T1(array[cluster])=[{"width"=424, "height"=240, "fps"=6, "Profile"=521292696, "ppx"=210.19093, "ppy"=123.56658, "fx"=317.53546, "fy"=317.53546, "model"=4}, {"width"=424, "height"=240, "fps"=15, "Profile"=521302424, "ppx"=210.19093, "ppy"=123.56658, "fx"=317.53546, "fy"=317.53546, "model"=4}, {"width"=424, "height"=240, "fps"=30, "Profile"=521300120, "ppx"=210.19093, "ppy"=123.56658, "fx"=317.53546, "fy"=317.53546, "model"=4}, {"width"=424, "height"=240, "fps"=60, "Profile"=521291928, "ppx"=210.19093, "ppy"=123.56658, "fx"=317.53546, "fy"=317.53546, "model"=4}, {"width"=424, "height"=240, "fps"=90, "Profile"=521301912, "ppx"=210.19093, "ppy"=123.56658, "fx"=317.53546, "fy"=317.53546, "model"=4}, {"width"=480, "height"=270, "fps"=6, "Profile"=521303704, "ppx"=237.96481, "ppy"=139.0124, "fx"=357.2274, "fy"=357.2274, "model"=4}, {"width"=480, "height"=270, "fps"=15, "Profile"=521304984, "ppx"=237.96481, "ppy"=139.0124, "fx"=357.2274, "fy"=357.2274, "model"=4}, {"width"=480, "height"=270, "fps"=30, "Profile"=521301144, "ppx"=237.96481, "ppy"=139.0124, "fx"=357.2274, "fy"=357.2274, "model"=4}, {"width"=480, "height"=270, "fps"=60, "Profile"=521300376, "ppx"=237.96481, "ppy"=139.0124, "fx"=357.2274, "fy"=357.2274, "model"=4}, {"width"=480, "height"=270, "fps"=90, "Profile"=521297560, "ppx"=237.96481, "ppy"=139.0124, "fx"=357.2274, "fy"=357.2274, "model"=4}, {"width"=640, "height"=360, "fps"=6, "Profile"=521313944, "ppx"=317.2864, "ppy"=185.34987, "fx"=476.3032, "fy"=476.3032, "model"=4}, {"width"=640, "height"=360, "fps"=15, "Profile"=521308312, "ppx"=317.2864, "ppy"=185.34987, "fx"=476.3032, "fy"=476.3032, "model"=4}, {"width"=640, "height"=360, "fps"=30, "Profile"=521293720, "ppx"=317.2864, "ppy"=185.34987, "fx"=476.3032, "fy"=476.3032, "model"=4}, {"width"=640, "height"=360, "fps"=60, "Profile"=521292952, "ppx"=317.2864, "ppy"=185.34987, "fx"=476.3032, "fy"=476.3032, "model"=4}, {"width"=640, "height"=360, "fps"=90, "Profile"=521306520, "ppx"=317.2864, "ppy"=185.34987, "fx"=476.3032, "fy"=476.3032, "model"=4}, {"width"=640, "height"=480, "fps"=6, "Profile"=521307800, "ppx"=316.38187, "ppy"=247.13316, "fx"=635.0709, "fy"=635.0709, "model"=4}, {"width"=640, "height"=480, "fps"=15, "Profile"=521316760, "ppx"=316.38187, "ppy"=247.13316, "fx"=635.0709, "fy"=635.0709, "model"=4}, {"width"=640, "height"=480, "fps"=30, "Profile"=521309848, "ppx"=316.38187, "ppy"=247.13316, "fx"=635.0709, "fy"=635.0709, "model"=4}, {"width"=640, "height"=480, "fps"=60, "Profile"=521318552, "ppx"=316.38187, "ppy"=247.13316, "fx"=635.0709, "fy"=635.0709, "model"=4}, {"width"=640, "height"=480, "fps"=90, "Profile"=521313432, "ppx"=316.38187, "ppy"=247.13316, "fx"=635.0709, "fy"=635.0709, "model"=4}, {"width"=848, "height"=480, "fps"=6, "Profile"=521308824, "ppx"=420.38187, "ppy"=247.13316, "fx"=635.0709, "fy"=635.0709, "model"=4}, {"width"=848, "height"=480, "fps"=15, "Profile"=521308056, "ppx"=420.38187, "ppy"=247.13316, "fx"=635.0709, "fy"=635.0709, "model"=4}, {"width"=848, "height"=480, "fps"=30, "Profile"=521320856, "ppx"=420.38187, "ppy"=247.13316, "fx"=635.0709, "fy"=635.0709, "model"=4}, {"width"=848, "height"=480, "fps"=60, "Profile"=521318040, "ppx"=420.38187, "ppy"=247.13316, "fx"=635.0709, "fy"=635.0709, "model"=4}, {"width"=848, "height"=480, "fps"=90, "Profile"=521322392, "ppx"=420.38187, "ppy"=247.13316, "fx"=635.0709, "fy"=635.0709, "model"=4}, {"width"=1280, "height"=720, "fps"=6, "Profile"=521315224, "ppx"=634.5728, "ppy"=370.69974, "fx"=952.6064, "fy"=952.6064, "model"=4}, {"width"=1280, "height"=720, "fps"=15, "Profile"=521316248, "ppx"=634.5728, "ppy"=370.69974, "fx"=952.6064, "fy"=952.6064, "model"=4}, {"width"=1280, "height"=720, "fps"=30, "Profile"=521319832, "ppx"=634.5728, "ppy"=370.69974, "fx"=952.6064, "fy"=952.6064, "model"=4}], 12 "IR left":T1(array[cluster])=[{"width"=424, "height"=240, "fps"=6, "Profile"=521311384, "ppx"=210.19093, "ppy"=123.56658, "fx"=317.53546, "fy"=317.53546, "model"=4}, {"width"=424, "height"=240, "fps"=15, "Profile"=521310104, "ppx"=210.19093, "ppy"=123.56658, "fx"=317.53546, "fy"=317.53546, "model"=4}, {"width"=424, "height"=240, "fps"=30, "Profile"=521314712, "ppx"=210.19093, "ppy"=123.56658, "fx"=317.53546, "fy"=317.53546, "model"=4}, {"width"=424, "height"=240, "fps"=60, "Profile"=521313688, "ppx"=210.19093, "ppy"=123.56658, "fx"=317.53546, "fy"=317.53546, "model"=4}, {"width"=424, "height"=240, "fps"=90, "Profile"=521315736, "ppx"=210.19093, "ppy"=123.56658, "fx"=317.53546, "fy"=317.53546, "model"=4}, {"width"=480, "height"=270, "fps"=6, "Profile"=521314968, "ppx"=237.96481, "ppy"=139.0124, "fx"=357.2274, "fy"=357.2274, "model"=4}, {"width"=480, "height"=270, "fps"=15, "Profile"=521318808, "ppx"=237.96481, "ppy"=139.0124, "fx"=357.2274, "fy"=357.2274, "model"=4}, {"width"=480, "height"=270, "fps"=30, "Profile"=521316504, "ppx"=237.96481, "ppy"=139.0124, "fx"=357.2274, "fy"=357.2274, "model"=4}, {"width"=480, "height"=270, "fps"=60, "Profile"=521322904, "ppx"=237.96481, "ppy"=139.0124, "fx"=357.2274, "fy"=357.2274, "model"=4}, {"width"=480, "height"=270, "fps"=90, "Profile"=521312152, "ppx"=237.96481, "ppy"=139.0124, "fx"=357.2274, "fy"=357.2274, "model"=4}, {"width"=640, "height"=360, "fps"=6, "Profile"=521314200, "ppx"=317.2864, "ppy"=185.34987, "fx"=476.3032, "fy"=476.3032, "model"=4}, {"width"=640, "height"=360, "fps"=15, "Profile"=521319320, "ppx"=317.2864, "ppy"=185.34987, "fx"=476.3032, "fy"=476.3032, "model"=4}, {"width"=640, "height"=360, "fps"=30, "Profile"=521319064, "ppx"=317.2864, "ppy"=185.34987, "fx"=476.3032, "fy"=476.3032, "model"=4}, {"width"=640, "height"=360, "fps"=60, "Profile"=521321112, "ppx"=317.2864, "ppy"=185.34987, "fx"=476.3032, "fy"=476.3032, "model"=4}, {"width"=640, "height"=360, "fps"=90, "Profile"=521318296, "ppx"=317.2864, "ppy"=185.34987, "fx"=476.3032, "fy"=476.3032, "model"=4}, {"width"=640, "height"=480, "fps"=6, "Profile"=521313176, "ppx"=316.38187, "ppy"=247.13316, "fx"=635.0709, "fy"=635.0709, "model"=4}, {"width"=640, "height"=480, "fps"=15, "Profile"=521321368, "ppx"=316.38187, "ppy"=247.13316, "fx"=635.0709, "fy"=635.0709, "model"=4}, {"width"=640, "height"=480, "fps"=30, "Profile"=521309592, "ppx"=316.38187, "ppy"=247.13316, "fx"=635.0709, "fy"=635.0709, "model"=4}, {"width"=640, "height"=480, "fps"=60, "Profile"=521320088, "ppx"=316.38187, "ppy"=247.13316, "fx"=635.0709, "fy"=635.0709, "model"=4}, {"width"=640, "height"=480, "fps"=90, "Profile"=521322648, "ppx"=316.38187, "ppy"=247.13316, "fx"=635.0709, "fy"=635.0709, "model"=4}, {"width"=848, "height"=480, "fps"=6, "Profile"=521315992, "ppx"=420.38187, "ppy"=247.13316, "fx"=635.0709, "fy"=635.0709, "model"=4}, {"width"=848, "height"=480, "fps"=15, "Profile"=521317272, "ppx"=420.38187, "ppy"=247.13316, "fx"=635.0709, "fy"=635.0709, "model"=4}, {"width"=848, "height"=480, "fps"=30, "Profile"=521310616, "ppx"=420.38187, "ppy"=247.13316, "fx"=635.0709, "fy"=635.0709, "model"=4}, {"width"=848, "height"=480, "fps"=60, "Profile"=521310360, "ppx"=420.38187, "ppy"=247.13316, "fx"=635.0709, "fy"=635.0709, "model"=4}, {"width"=848, "height"=480, "fps"=90, "Profile"=521306776, "ppx"=420.38187, "ppy"=247.13316, "fx"=635.0709, "fy"=635.0709, "model"=4}, {"width"=1280, "height"=720, "fps"=6, "Profile"=521320600, "ppx"=634.5728, "ppy"=370.69974, "fx"=952.6064, "fy"=952.6064, "model"=4}, {"width"=1280, "height"=720, "fps"=15, "Profile"=521310872, "ppx"=634.5728, "ppy"=370.69974, "fx"=952.6064, "fy"=952.6064, "model"=4}, {"width"=1280, "height"=720, "fps"=30, "Profile"=521320344, "ppx"=634.5728, "ppy"=370.69974, "fx"=952.6064, "fy"=952.6064, "model"=4}, {"width"=1920, "height"=1080, "fps"=15, "Profile"=521627576, "ppx"=951.85925, "ppy"=556.0496, "fx"=1428.9095, "fy"=1428.9095, "model"=4}, {"width"=1920, "height"=1080, "fps"=25, "Profile"=521617080, "ppx"=951.85925, "ppy"=556.0496, "fx"=1428.9095, "fy"=1428.9095, "model"=4}], 13 "IR Right":T1(array[cluster])=[{"width"=424, "height"=240, "fps"=6, "Profile"=521602232, "ppx"=210.19093, "ppy"=123.56658, "fx"=317.53546, "fy"=317.53546, "model"=4}, {"width"=424, "height"=240, "fps"=15, "Profile"=521611192, "ppx"=210.19093, "ppy"=123.56658, "fx"=317.53546, "fy"=317.53546, "model"=4}, {"width"=424, "height"=240, "fps"=30, "Profile"=521614264, "ppx"=210.19093, "ppy"=123.56658, "fx"=317.53546, "fy"=317.53546, "model"=4}, {"width"=424, "height"=240, "fps"=60, "Profile"=521614008, "ppx"=210.19093, "ppy"=123.56658, "fx"=317.53546, "fy"=317.53546, "model"=4}, {"width"=424, "height"=240, "fps"=90, "Profile"=521601976, "ppx"=210.19093, "ppy"=123.56658, "fx"=317.53546, "fy"=317.53546, "model"=4}, {"width"=480, "height"=270, "fps"=6, "Profile"=521602488, "ppx"=237.96481, "ppy"=139.0124, "fx"=357.2274, "fy"=357.2274, "model"=4}, {"width"=480, "height"=270, "fps"=15, "Profile"=521610936, "ppx"=237.96481, "ppy"=139.0124, "fx"=357.2274, "fy"=357.2274, "model"=4}, {"width"=480, "height"=270, "fps"=30, "Profile"=521605048, "ppx"=237.96481, "ppy"=139.0124, "fx"=357.2274, "fy"=357.2274, "model"=4}, {"width"=480, "height"=270, "fps"=60, "Profile"=521603000, "ppx"=237.96481, "ppy"=139.0124, "fx"=357.2274, "fy"=357.2274, "model"=4}, {"width"=480, "height"=270, "fps"=90, "Profile"=521612216, "ppx"=237.96481, "ppy"=139.0124, "fx"=357.2274, "fy"=357.2274, "model"=4}, {"width"=640, "height"=360, "fps"=6, "Profile"=521611448, "ppx"=317.2864, "ppy"=185.34987, "fx"=476.3032, "fy"=476.3032, "model"=4}, {"width"=640, "height"=360, "fps"=15, "Profile"=521613496, "ppx"=317.2864, "ppy"=185.34987, "fx"=476.3032, "fy"=476.3032, "model"=4}, {"width"=640, "height"=360, "fps"=30, "Profile"=521604792, "ppx"=317.2864, "ppy"=185.34987, "fx"=476.3032, "fy"=476.3032, "model"=4}, {"width"=640, "height"=360, "fps"=60, "Profile"=521606072, "ppx"=317.2864, "ppy"=185.34987, "fx"=476.3032, "fy"=476.3032, "model"=4}, {"width"=640, "height"=360, "fps"=90, "Profile"=521609656, "ppx"=317.2864, "ppy"=185.34987, "fx"=476.3032, "fy"=476.3032, "model"=4}, {"width"=640, "height"=480, "fps"=6, "Profile"=521608376, "ppx"=316.38187, "ppy"=247.13316, "fx"=635.0709, "fy"=635.0709, "model"=4}, {"width"=640, "height"=480, "fps"=15, "Profile"=521608120, "ppx"=316.38187, "ppy"=247.13316, "fx"=635.0709, "fy"=635.0709, "model"=4}, {"width"=640, "height"=480, "fps"=30, "Profile"=521607352, "ppx"=316.38187, "ppy"=247.13316, "fx"=635.0709, "fy"=635.0709, "model"=4}, {"width"=640, "height"=480, "fps"=60, "Profile"=521615032, "ppx"=316.38187, "ppy"=247.13316, "fx"=635.0709, "fy"=635.0709, "model"=4}, {"width"=640, "height"=480, "fps"=90, "Profile"=521605304, "ppx"=316.38187, "ppy"=247.13316, "fx"=635.0709, "fy"=635.0709, "model"=4}, {"width"=848, "height"=480, "fps"=6, "Profile"=521616568, "ppx"=420.38187, "ppy"=247.13316, "fx"=635.0709, "fy"=635.0709, "model"=4}, {"width"=848, "height"=480, "fps"=15, "Profile"=521615288, "ppx"=420.38187, "ppy"=247.13316, "fx"=635.0709, "fy"=635.0709, "model"=4}, {"width"=848, "height"=480, "fps"=30, "Profile"=521609144, "ppx"=420.38187, "ppy"=247.13316, "fx"=635.0709, "fy"=635.0709, "model"=4}, {"width"=848, "height"=480, "fps"=60, "Profile"=521611960, "ppx"=420.38187, "ppy"=247.13316, "fx"=635.0709, "fy"=635.0709, "model"=4}, {"width"=848, "height"=480, "fps"=90, "Profile"=521614776, "ppx"=420.38187, "ppy"=247.13316, "fx"=635.0709, "fy"=635.0709, "model"=4}, {"width"=1280, "height"=720, "fps"=6, "Profile"=521608888, "ppx"=634.5728, "ppy"=370.69974, "fx"=952.6064, "fy"=952.6064, "model"=4}, {"width"=1280, "height"=720, "fps"=15, "Profile"=521616824, "ppx"=634.5728, "ppy"=370.69974, "fx"=952.6064, "fy"=952.6064, "model"=4}, {"width"=1280, "height"=720, "fps"=30, "Profile"=521615544, "ppx"=634.5728, "ppy"=370.69974, "fx"=952.6064, "fy"=952.6064, "model"=4}, {"width"=1920, "height"=1080, "fps"=15, "Profile"=521628088, "ppx"=951.85925, "ppy"=556.0496, "fx"=1428.9095, "fy"=1428.9095, "model"=4}, {"width"=1920, "height"=1080, "fps"=25, "Profile"=521608632, "ppx"=951.85925, "ppy"=556.0496, "fx"=1428.9095, "fy"=1428.9095, "model"=4}], 14 "Depth Stream":T1(array[cluster])=[{"width"=424, "height"=240, "fps"=6, "Profile"=521292696, "ppx"=210.19093, "ppy"=123.56658, "fx"=317.53546, "fy"=317.53546, "model"=4}, {"width"=424, "height"=240, "fps"=15, "Profile"=521302424, "ppx"=210.19093, "ppy"=123.56658, "fx"=317.53546, "fy"=317.53546, "model"=4}, {"width"=424, "height"=240, "fps"=30, "Profile"=521300120, "ppx"=210.19093, "ppy"=123.56658, "fx"=317.53546, "fy"=317.53546, "model"=4}, {"width"=424, "height"=240, "fps"=60, "Profile"=521291928, "ppx"=210.19093, "ppy"=123.56658, "fx"=317.53546, "fy"=317.53546, "model"=4}, {"width"=424, "height"=240, "fps"=90, "Profile"=521301912, "ppx"=210.19093, "ppy"=123.56658, "fx"=317.53546, "fy"=317.53546, "model"=4}, {"width"=480, "height"=270, "fps"=6, "Profile"=521303704, "ppx"=237.96481, "ppy"=139.0124, "fx"=357.2274, "fy"=357.2274, "model"=4}, {"width"=480, "height"=270, "fps"=15, "Profile"=521304984, "ppx"=237.96481, "ppy"=139.0124, "fx"=357.2274, "fy"=357.2274, "model"=4}, {"width"=480, "height"=270, "fps"=30, "Profile"=521301144, "ppx"=237.96481, "ppy"=139.0124, "fx"=357.2274, "fy"=357.2274, "model"=4}, {"width"=480, "height"=270, "fps"=60, "Profile"=521300376, "ppx"=237.96481, "ppy"=139.0124, "fx"=357.2274, "fy"=357.2274, "model"=4}, {"width"=480, "height"=270, "fps"=90, "Profile"=521297560, "ppx"=237.96481, "ppy"=139.0124, "fx"=357.2274, "fy"=357.2274, "model"=4}, {"width"=640, "height"=360, "fps"=6, "Profile"=521313944, "ppx"=317.2864, "ppy"=185.34987, "fx"=476.3032, "fy"=476.3032, "model"=4}, {"width"=640, "height"=360, "fps"=15, "Profile"=521308312, "ppx"=317.2864, "ppy"=185.34987, "fx"=476.3032, "fy"=476.3032, "model"=4}, {"width"=640, "height"=360, "fps"=30, "Profile"=521293720, "ppx"=317.2864, "ppy"=185.34987, "fx"=476.3032, "fy"=476.3032, "model"=4}, {"width"=640, "height"=360, "fps"=60, "Profile"=521292952, "ppx"=317.2864, "ppy"=185.34987, "fx"=476.3032, "fy"=476.3032, "model"=4}, {"width"=640, "height"=360, "fps"=90, "Profile"=521306520, "ppx"=317.2864, "ppy"=185.34987, "fx"=476.3032, "fy"=476.3032, "model"=4}, {"width"=640, "height"=480, "fps"=6, "Profile"=521307800, "ppx"=316.38187, "ppy"=247.13316, "fx"=635.0709, "fy"=635.0709, "model"=4}, {"width"=640, "height"=480, "fps"=15, "Profile"=521316760, "ppx"=316.38187, "ppy"=247.13316, "fx"=635.0709, "fy"=635.0709, "model"=4}, {"width"=640, "height"=480, "fps"=30, "Profile"=521309848, "ppx"=316.38187, "ppy"=247.13316, "fx"=635.0709, "fy"=635.0709, "model"=4}, {"width"=640, "height"=480, "fps"=60, "Profile"=521318552, "ppx"=316.38187, "ppy"=247.13316, "fx"=635.0709, "fy"=635.0709, "model"=4}, {"width"=640, "height"=480, "fps"=90, "Profile"=521313432, "ppx"=316.38187, "ppy"=247.13316, "fx"=635.0709, "fy"=635.0709, "model"=4}, {"width"=848, "height"=480, "fps"=6, "Profile"=521308824, "ppx"=420.38187, "ppy"=247.13316, "fx"=635.0709, "fy"=635.0709, "model"=4}, {"width"=848, "height"=480, "fps"=15, "Profile"=521308056, "ppx"=420.38187, "ppy"=247.13316, "fx"=635.0709, "fy"=635.0709, "model"=4}, {"width"=848, "height"=480, "fps"=30, "Profile"=521320856, "ppx"=420.38187, "ppy"=247.13316, "fx"=635.0709, "fy"=635.0709, "model"=4}, {"width"=848, "height"=480, "fps"=60, "Profile"=521318040, "ppx"=420.38187, "ppy"=247.13316, "fx"=635.0709, "fy"=635.0709, "model"=4}, {"width"=848, "height"=480, "fps"=90, "Profile"=521322392, "ppx"=420.38187, "ppy"=247.13316, "fx"=635.0709, "fy"=635.0709, "model"=4}, {"width"=1280, "height"=720, "fps"=6, "Profile"=521315224, "ppx"=634.5728, "ppy"=370.69974, "fx"=952.6064, "fy"=952.6064, "model"=4}, {"width"=1280, "height"=720, "fps"=15, "Profile"=521316248, "ppx"=634.5728, "ppy"=370.69974, "fx"=952.6064, "fy"=952.6064, "model"=4}, {"width"=1280, "height"=720, "fps"=30, "Profile"=521319832, "ppx"=634.5728, "ppy"=370.69974, "fx"=952.6064, "fy"=952.6064, "model"=4}], 15 "Depth Stream strings":string[](array[string])=["424 x 240 @6fps", "424 x 240 @15fps", "424 x 240 @30fps", "424 x 240 @60fps", "424 x 240 @90fps", "480 x 270 @6fps", "480 x 270 @15fps", "480 x 270 @30fps", "480 x 270 @60fps", "480 x 270 @90fps", "640 x 360 @6fps", "640 x 360 @15fps", "640 x 360 @30fps", "640 x 360 @60fps", "640 x 360 @90fps", "640 x 480 @6fps", "640 x 480 @15fps", "640 x 480 @30fps", "640 x 480 @60fps", "640 x 480 @90fps", "848 x 480 @6fps", "848 x 480 @15fps", "848 x 480 @30fps", "848 x 480 @60fps", "848 x 480 @90fps", "1280 x 720 @6fps", "1280 x 720 @15fps", "1280 x 720 @30fps"], 16 "Depth Stream strings Compress":string[](array[string])=["424 x 240 @6fps", "424 x 240 @15fps", "424 x 240 @30fps", "424 x 240 @60fps", "424 x 240 @90fps", "480 x 270 @6fps", "480 x 270 @15fps", "480 x 270 @30fps", "480 x 270 @60fps", "480 x 270 @90fps", "640 x 360 @6fps", "640 x 360 @15fps", "640 x 360 @30fps", "640 x 360 @60fps", "640 x 360 @90fps", "640 x 480 @6fps", "640 x 480 @15fps", "640 x 480 @30fps", "640 x 480 @60fps", "640 x 480 @90fps", "848 x 480 @6fps", "848 x 480 @15fps", "848 x 480 @30fps", "848 x 480 @60fps", "848 x 480 @90fps", "1280 x 720 @6fps", "1280 x 720 @15fps", "1280 x 720 @30fps"], 17 "Depth Stream Compress.":T1(array[cluster])=[{"width"=424, "height"=240, "fps"=6, "Profile"=521292696, "ppx"=210.19093, "ppy"=123.56658, "fx"=317.53546, "fy"=317.53546, "model"=4}, {"width"=424, "height"=240, "fps"=15, "Profile"=521302424, "ppx"=210.19093, "ppy"=123.56658, "fx"=317.53546, "fy"=317.53546, "model"=4}, {"width"=424, "height"=240, "fps"=30, "Profile"=521300120, "ppx"=210.19093, "ppy"=123.56658, "fx"=317.53546, "fy"=317.53546, "model"=4}, {"width"=424, "height"=240, "fps"=60, "Profile"=521291928, "ppx"=210.19093, "ppy"=123.56658, "fx"=317.53546, "fy"=317.53546, "model"=4}, {"width"=424, "height"=240, "fps"=90, "Profile"=521301912, "ppx"=210.19093, "ppy"=123.56658, "fx"=317.53546, "fy"=317.53546, "model"=4}, {"width"=480, "height"=270, "fps"=6, "Profile"=521303704, "ppx"=237.96481, "ppy"=139.0124, "fx"=357.2274, "fy"=357.2274, "model"=4}, {"width"=480, "height"=270, "fps"=15, "Profile"=521304984, "ppx"=237.96481, "ppy"=139.0124, "fx"=357.2274, "fy"=357.2274, "model"=4}, {"width"=480, "height"=270, "fps"=30, "Profile"=521301144, "ppx"=237.96481, "ppy"=139.0124, "fx"=357.2274, "fy"=357.2274, "model"=4}, {"width"=480, "height"=270, "fps"=60, "Profile"=521300376, "ppx"=237.96481, "ppy"=139.0124, "fx"=357.2274, "fy"=357.2274, "model"=4}, {"width"=480, "height"=270, "fps"=90, "Profile"=521297560, "ppx"=237.96481, "ppy"=139.0124, "fx"=357.2274, "fy"=357.2274, "model"=4}, {"width"=640, "height"=360, "fps"=6, "Profile"=521313944, "ppx"=317.2864, "ppy"=185.34987, "fx"=476.3032, "fy"=476.3032, "model"=4}, {"width"=640, "height"=360, "fps"=15, "Profile"=521308312, "ppx"=317.2864, "ppy"=185.34987, "fx"=476.3032, "fy"=476.3032, "model"=4}, {"width"=640, "height"=360, "fps"=30, "Profile"=521293720, "ppx"=317.2864, "ppy"=185.34987, "fx"=476.3032, "fy"=476.3032, "model"=4}, {"width"=640, "height"=360, "fps"=60, "Profile"=521292952, "ppx"=317.2864, "ppy"=185.34987, "fx"=476.3032, "fy"=476.3032, "model"=4}, {"width"=640, "height"=360, "fps"=90, "Profile"=521306520, "ppx"=317.2864, "ppy"=185.34987, "fx"=476.3032, "fy"=476.3032, "model"=4}, {"width"=640, "height"=480, "fps"=6, "Profile"=521307800, "ppx"=316.38187, "ppy"=247.13316, "fx"=635.0709, "fy"=635.0709, "model"=4}, {"width"=640, "height"=480, "fps"=15, "Profile"=521316760, "ppx"=316.38187, "ppy"=247.13316, "fx"=635.0709, "fy"=635.0709, "model"=4}, {"width"=640, "height"=480, "fps"=30, "Profile"=521309848, "ppx"=316.38187, "ppy"=247.13316, "fx"=635.0709, "fy"=635.0709, "model"=4}, {"width"=640, "height"=480, "fps"=60, "Profile"=521318552, "ppx"=316.38187, "ppy"=247.13316, "fx"=635.0709, "fy"=635.0709, "model"=4}, {"width"=640, "height"=480, "fps"=90, "Profile"=521313432, "ppx"=316.38187, "ppy"=247.13316, "fx"=635.0709, "fy"=635.0709, "model"=4}, {"width"=848, "height"=480, "fps"=6, "Profile"=521308824, "ppx"=420.38187, "ppy"=247.13316, "fx"=635.0709, "fy"=635.0709, "model"=4}, {"width"=848, "height"=480, "fps"=15, "Profile"=521308056, "ppx"=420.38187, "ppy"=247.13316, "fx"=635.0709, "fy"=635.0709, "model"=4}, {"width"=848, "height"=480, "fps"=30, "Profile"=521320856, "ppx"=420.38187, "ppy"=247.13316, "fx"=635.0709, "fy"=635.0709, "model"=4}, {"width"=848, "height"=480, "fps"=60, "Profile"=521318040, "ppx"=420.38187, "ppy"=247.13316, "fx"=635.0709, "fy"=635.0709, "model"=4}, {"width"=848, "height"=480, "fps"=90, "Profile"=521322392, "ppx"=420.38187, "ppy"=247.13316, "fx"=635.0709, "fy"=635.0709, "model"=4}, {"width"=1280, "height"=720, "fps"=6, "Profile"=521315224, "ppx"=634.5728, "ppy"=370.69974, "fx"=952.6064, "fy"=952.6064, "model"=4}, {"width"=1280, "height"=720, "fps"=15, "Profile"=521316248, "ppx"=634.5728, "ppy"=370.69974, "fx"=952.6064, "fy"=952.6064, "model"=4}, {"width"=1280, "height"=720, "fps"=30, "Profile"=521319832, "ppx"=634.5728, "ppy"=370.69974, "fx"=952.6064, "fy"=952.6064, "model"=4}], 18 "Color Left":T1(array[cluster])=[{"width"=424, "height"=240, "fps"=6, "Profile"=521327256, "ppx"=210.19093, "ppy"=123.56658, "fx"=317.53546, "fy"=317.53546, "model"=4}, {"width"=424, "height"=240, "fps"=15, "Profile"=521335960, "ppx"=210.19093, "ppy"=123.56658, "fx"=317.53546, "fy"=317.53546, "model"=4}, {"width"=424, "height"=240, "fps"=30, "Profile"=521336216, "ppx"=210.19093, "ppy"=123.56658, "fx"=317.53546, "fy"=317.53546, "model"=4}, {"width"=424, "height"=240, "fps"=60, "Profile"=521334936, "ppx"=210.19093, "ppy"=123.56658, "fx"=317.53546, "fy"=317.53546, "model"=4}, {"width"=424, "height"=240, "fps"=90, "Profile"=521321624, "ppx"=210.19093, "ppy"=123.56658, "fx"=317.53546, "fy"=317.53546, "model"=4}, {"width"=480, "height"=270, "fps"=6, "Profile"=521329048, "ppx"=237.96481, "ppy"=139.0124, "fx"=357.2274, "fy"=357.2274, "model"=4}, {"width"=480, "height"=270, "fps"=15, "Profile"=521323672, "ppx"=237.96481, "ppy"=139.0124, "fx"=357.2274, "fy"=357.2274, "model"=4}, {"width"=480, "height"=270, "fps"=30, "Profile"=521332632, "ppx"=237.96481, "ppy"=139.0124, "fx"=357.2274, "fy"=357.2274, "model"=4}, {"width"=480, "height"=270, "fps"=60, "Profile"=521337496, "ppx"=237.96481, "ppy"=139.0124, "fx"=357.2274, "fy"=357.2274, "model"=4}, {"width"=480, "height"=270, "fps"=90, "Profile"=521326232, "ppx"=237.96481, "ppy"=139.0124, "fx"=357.2274, "fy"=357.2274, "model"=4}, {"width"=640, "height"=360, "fps"=6, "Profile"=521353112, "ppx"=317.2864, "ppy"=185.34987, "fx"=476.3032, "fy"=476.3032, "model"=4}, {"width"=640, "height"=360, "fps"=15, "Profile"=521347992, "ppx"=317.2864, "ppy"=185.34987, "fx"=476.3032, "fy"=476.3032, "model"=4}, {"width"=640, "height"=360, "fps"=30, "Profile"=521345432, "ppx"=317.2864, "ppy"=185.34987, "fx"=476.3032, "fy"=476.3032, "model"=4}, {"width"=640, "height"=360, "fps"=60, "Profile"=521332888, "ppx"=317.2864, "ppy"=185.34987, "fx"=476.3032, "fy"=476.3032, "model"=4}, {"width"=640, "height"=360, "fps"=90, "Profile"=521326744, "ppx"=317.2864, "ppy"=185.34987, "fx"=476.3032, "fy"=476.3032, "model"=4}, {"width"=640, "height"=480, "fps"=6, "Profile"=521349272, "ppx"=316.38187, "ppy"=247.13316, "fx"=635.0709, "fy"=635.0709, "model"=4}, {"width"=640, "height"=480, "fps"=15, "Profile"=521350808, "ppx"=316.38187, "ppy"=247.13316, "fx"=635.0709, "fy"=635.0709, "model"=4}, {"width"=640, "height"=480, "fps"=30, "Profile"=521350296, "ppx"=316.38187, "ppy"=247.13316, "fx"=635.0709, "fy"=635.0709, "model"=4}, {"width"=640, "height"=480, "fps"=60, "Profile"=521345944, "ppx"=316.38187, "ppy"=247.13316, "fx"=635.0709, "fy"=635.0709, "model"=4}, {"width"=640, "height"=480, "fps"=90, "Profile"=521351576, "ppx"=316.38187, "ppy"=247.13316, "fx"=635.0709, "fy"=635.0709, "model"=4}, {"width"=848, "height"=480, "fps"=6, "Profile"=521610680, "ppx"=420.38187, "ppy"=247.13316, "fx"=635.0709, "fy"=635.0709, "model"=4}, {"width"=848, "height"=480, "fps"=15, "Profile"=521617592, "ppx"=420.38187, "ppy"=247.13316, "fx"=635.0709, "fy"=635.0709, "model"=4}, {"width"=848, "height"=480, "fps"=30, "Profile"=521343640, "ppx"=420.38187, "ppy"=247.13316, "fx"=635.0709, "fy"=635.0709, "model"=4}, {"width"=848, "height"=480, "fps"=60, "Profile"=521354136, "ppx"=420.38187, "ppy"=247.13316, "fx"=635.0709, "fy"=635.0709, "model"=4}, {"width"=848, "height"=480, "fps"=90, "Profile"=521351064, "ppx"=420.38187, "ppy"=247.13316, "fx"=635.0709, "fy"=635.0709, "model"=4}, {"width"=1280, "height"=720, "fps"=6, "Profile"=521617336, "ppx"=634.5728, "ppy"=370.69974, "fx"=952.6064, "fy"=952.6064, "model"=4}, {"width"=1280, "height"=720, "fps"=15, "Profile"=521604536, "ppx"=634.5728, "ppy"=370.69974, "fx"=952.6064, "fy"=952.6064, "model"=4}, {"width"=1280, "height"=720, "fps"=30, "Profile"=521605560, "ppx"=634.5728, "ppy"=370.69974, "fx"=952.6064, "fy"=952.6064, "model"=4}], 19 "Color Left Array":string[](array[string])=["424 x 240 @6fps", "424 x 240 @15fps", "424 x 240 @30fps", "424 x 240 @60fps", "424 x 240 @90fps", "480 x 270 @6fps", "480 x 270 @15fps", "480 x 270 @30fps", "480 x 270 @60fps", "480 x 270 @90fps", "640 x 360 @6fps", "640 x 360 @15fps", "640 x 360 @30fps", "640 x 360 @60fps", "640 x 360 @90fps", "640 x 480 @6fps", "640 x 480 @15fps", "640 x 480 @30fps", "640 x 480 @60fps", "640 x 480 @90fps", "848 x 480 @6fps", "848 x 480 @15fps", "848 x 480 @30fps", "848 x 480 @60fps", "848 x 480 @90fps", "1280 x 720 @6fps", "1280 x 720 @15fps", "1280 x 720 @30fps"])   [LabVIEW 2017, in "libRealSense3.lvlib"]
doc: "This helper VI is used to decode the numerous streams, and parse them into arrays of Depth, Color Left, IR left, IR Right, Unrectified L, Unrectified R."
uses:
  libRealSense3.lvlib
panel:
  # "RS3 Decode Depth Streams"
  # "(C) Intel Corp.,  AGJ 2018"
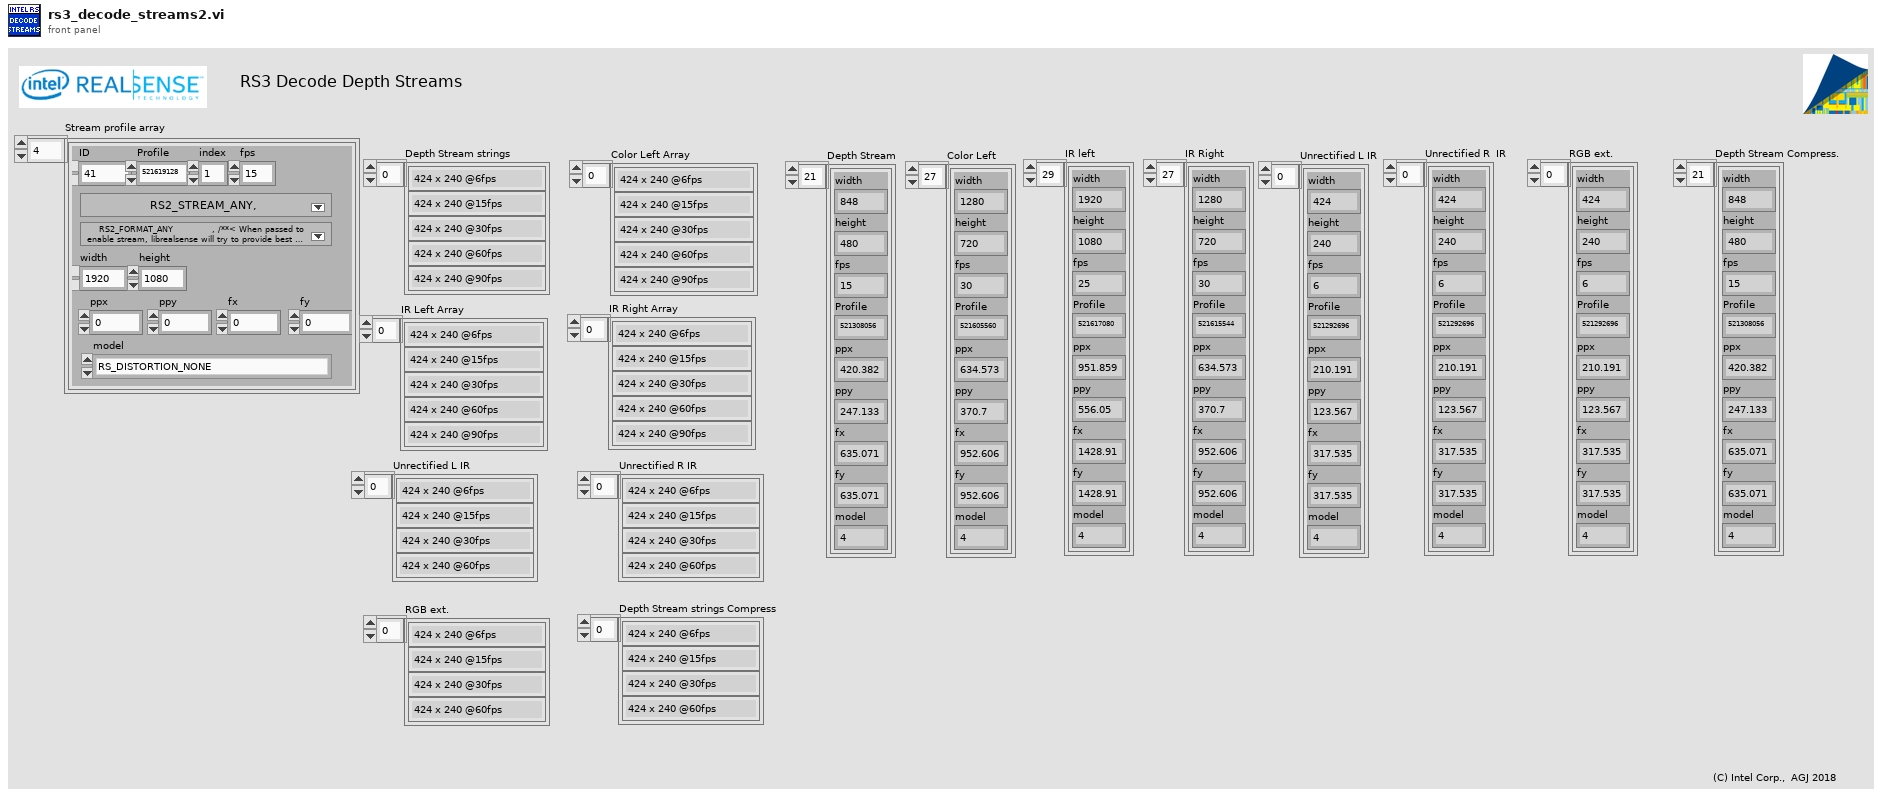
[diagram p1: front panel]
types:
  T1 = cluster{"width":i32, "height":i32, "fps":i32, "Profile":u64, "ppx":sgl, "ppy":sgl, "fx":sgl, "fy":sgl, "model":u32}[]
  T2 = cluster{"ID":i32, "Profile":u64, "fps":i32, "RS Stream":u16, "RS Format":u16, "index":u16, "width":i32, "height":i32, "ppx":sgl, "ppy":sgl, "fx":sgl, "fy":sgl, "model":u32}[]
  T3 = cluster{"width":i32, "height":i32, "fps":i32, "Profile":u64, "ppx":sgl, "ppy":sgl, "fx":sgl, "fy":sgl, "model":u32}
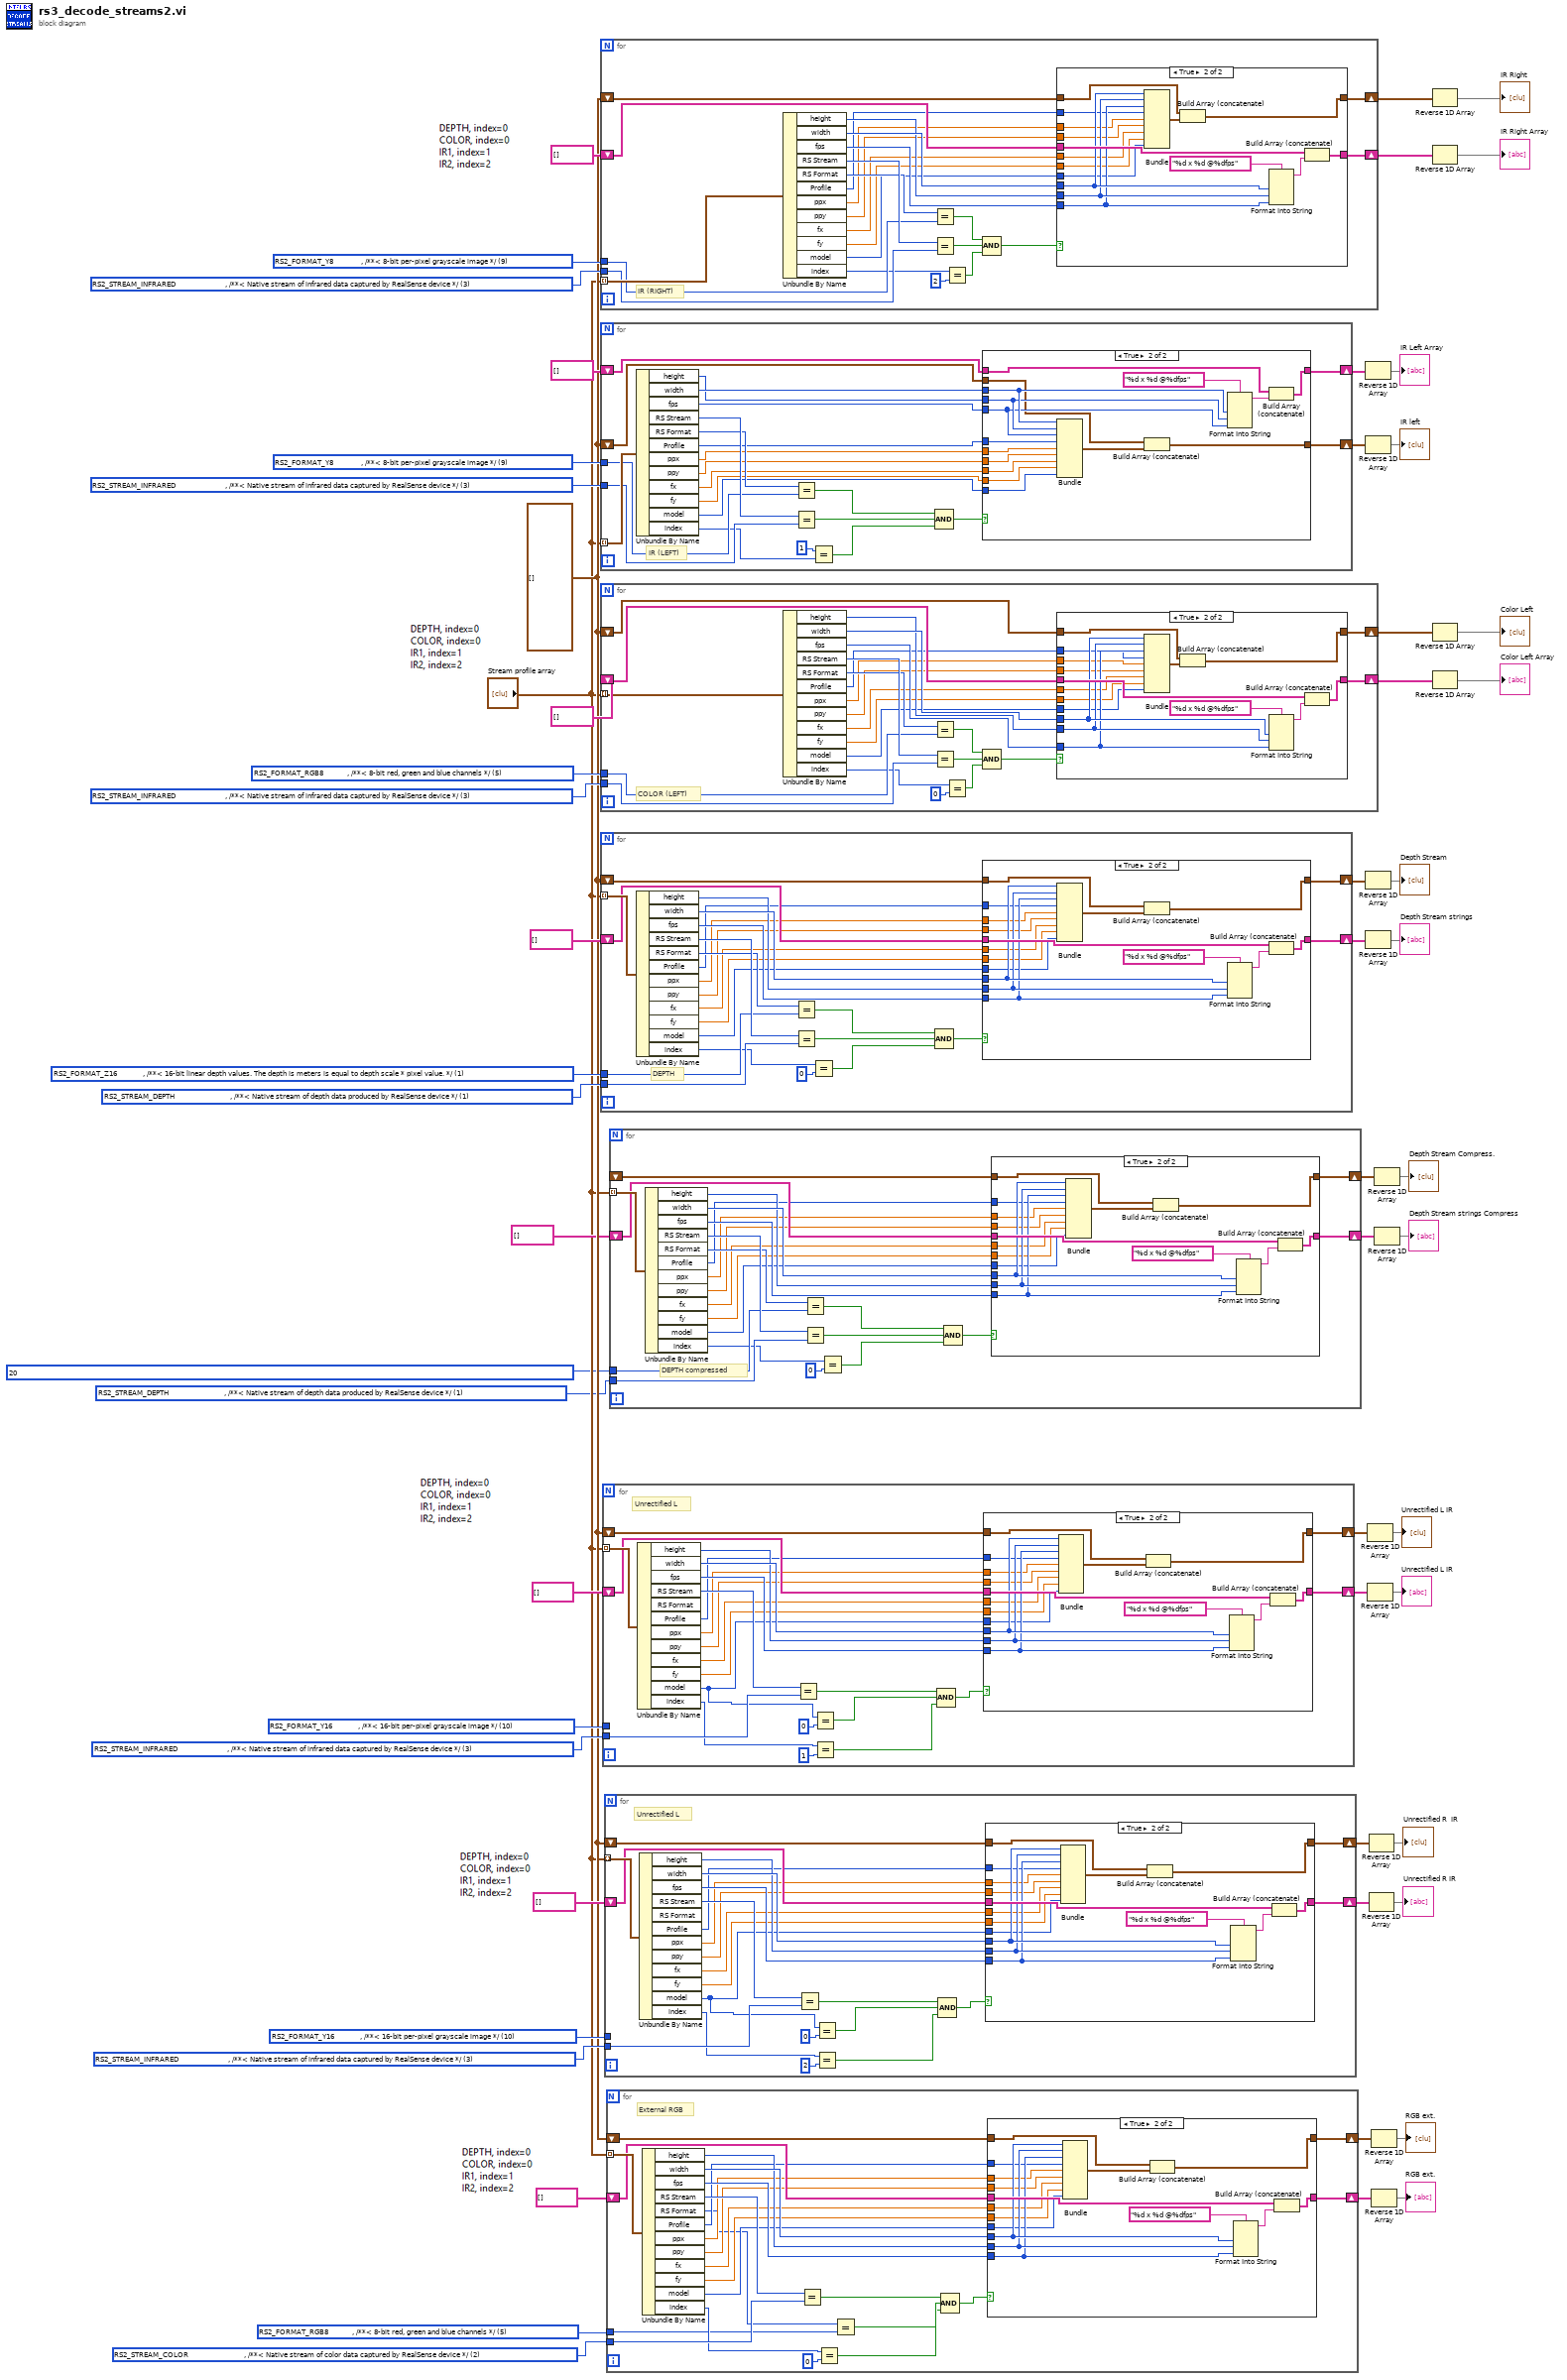
[diagram p0: block diagram]
diagram:
  w1 = u16 1 items=["    RS2_STREAM_ANY,", "    RS2_STREAM_DEPTH                            , /**< Native stream of depth data produced by RealSense device */", "    RS2_STREAM_COLOR                            , /**< Native stream of color data captured by RealSense device */", "    RS2_STREAM_INFRARED                         , /**< Native stream of infrared data captured by RealSense device */", "    RS2_STREAM_FISHEYE                          , /**< Native stream of fish-eye (wide) data captured from the dedicate motion camera */", "    RS2_STREAM_GYRO                             , /**< Native stream of gyroscope motion data produced by RealSense device */", "    RS2_STREAM_ACCEL                            , /**< Native stream of accelerometer motion data produced by RealSense device */", "    RS2_STREAM_GPIO                             , /**< Signals from external device connected through GPIO */", "    RS2_STREAM_POSE                             , /**< 6 Degrees of Freedom pose data, calculated by RealSense device */", "    RS2_STREAM_CONFIDENCE,", "    RS2_STREAM_COUNT"] ("RS Stream")
  w12 = u16 5 items=["    RS2_FORMAT_ANY             , /**< When passed to enable stream, librealsense will try to provide best suited format */", "    RS2_FORMAT_Z16             , /**< 16-bit linear depth values. The depth is meters is equal to depth scale * pixel value. */", "    RS2_FORMAT_DISPARITY16     , /**< 16-bit linear disparity values. The depth in meters is equal to depth scale / pixel value. */", "    RS2_FORMAT_XYZ32F          , /**< 32-bit floating point 3D coordinates. */", "    RS2_FORMAT_YUYV            , /**< Standard YUV pixel format as described in https://en.wikipedia.org/wiki/YUV */", "    RS2_FORMAT_RGB8            , /**< 8-bit red, green and blue channels */", "    RS2_FORMAT_BGR8            , /**< 8-bit blue, green, and red channels -- suitable for OpenCV */", "    RS2_FORMAT_RGBA8           , /**< 8-bit red, green and blue channels + constant alpha channel equal to FF */", "    RS2_FORMAT_BGRA8           , /**< 8-bit blue, green, and red channels + constant alpha channel equal to FF */", "    RS2_FORMAT_Y8              , /**< 8-bit per-pixel grayscale image */", "    RS2_FORMAT_Y16             , /**< 16-bit per-pixel grayscale image */", "    RS2_FORMAT_RAW10           , /**< Four 10-bit luminance values encoded into a 5-byte macropixel */", "    RS2_FORMAT_RAW16           , /**< 16-bit raw image */", "    RS2_FORMAT_RAW8            , /**< 8-bit raw image */", "    RS2_FORMAT_UYVY            , /**< Similar to the standard YUYV pixel format, but packed in a different order */", "    RS2_FORMAT_MOTION_RAW      , /**< Raw data from the motion sensor */", "    RS2_FORMAT_MOTION_XYZ32F   , /**< Motion data packed as 3 32-bit float values, for X, Y, and Z axis */", "    RS2_FORMAT_GPIO_RAW        , /**< Raw data from the external sensors hooked to one of the GPIO's */", "    RS2_FORMAT_COUNT             /**< Number of enumeration values. Not a valid input: intended to be used in for-loops. */"] ("RS Format")
  w11 = u16 2 items=["    RS2_STREAM_ANY,", "    RS2_STREAM_DEPTH                            , /**< Native stream of depth data produced by RealSense device */", "    RS2_STREAM_COLOR                            , /**< Native stream of color data captured by RealSense device */", "    RS2_STREAM_INFRARED                         , /**< Native stream of infrared data captured by RealSense device */", "    RS2_STREAM_FISHEYE                          , /**< Native stream of fish-eye (wide) data captured from the dedicate motion camera */", "    RS2_STREAM_GYRO                             , /**< Native stream of gyroscope motion data produced by RealSense device */", "    RS2_STREAM_ACCEL                            , /**< Native stream of accelerometer motion data produced by RealSense device */", "    RS2_STREAM_GPIO                             , /**< Signals from external device connected through GPIO */", "    RS2_STREAM_COUNT"] ("RS Stream")
  w24 = u16 10 items=["    RS2_FORMAT_ANY             , /**< When passed to enable stream, librealsense will try to provide best suited format */", "    RS2_FORMAT_Z16             , /**< 16-bit linear depth values. The depth is meters is equal to depth scale * pixel value. */", "    RS2_FORMAT_DISPARITY16     , /**< 16-bit linear disparity values. The depth in meters is equal to depth scale / pixel value. */", "    RS2_FORMAT_XYZ32F          , /**< 32-bit floating point 3D coordinates. */", "    RS2_FORMAT_YUYV            , /**< Standard YUV pixel format as described in https://en.wikipedia.org/wiki/YUV */", "    RS2_FORMAT_RGB8            , /**< 8-bit red, green and blue channels */", "    RS2_FORMAT_BGR8            , /**< 8-bit blue, green, and red channels -- suitable for OpenCV */", "    RS2_FORMAT_RGBA8           , /**< 8-bit red, green and blue channels + constant alpha channel equal to FF */", "    RS2_FORMAT_BGRA8           , /**< 8-bit blue, green, and red channels + constant alpha channel equal to FF */", "    RS2_FORMAT_Y8              , /**< 8-bit per-pixel grayscale image */", "    RS2_FORMAT_Y16             , /**< 16-bit per-pixel grayscale image */", "    RS2_FORMAT_RAW10           , /**< Four 10-bit luminance values encoded into a 5-byte macropixel */", "    RS2_FORMAT_RAW16           , /**< 16-bit raw image */", "    RS2_FORMAT_RAW8            , /**< 8-bit raw image */", "    RS2_FORMAT_UYVY            , /**< Similar to the standard YUYV pixel format, but packed in a different order */", "    RS2_FORMAT_MOTION_RAW      , /**< Raw data from the motion sensor */", "    RS2_FORMAT_MOTION_XYZ32F   , /**< Motion data packed as 3 32-bit float values, for X, Y, and Z axis */", "    RS2_FORMAT_GPIO_RAW        , /**< Raw data from the external sensors hooked to one of the GPIO's */", "    RS2_FORMAT_COUNT             /**< Number of enumeration values. Not a valid input: intended to be used in for-loops. */"] ("RS Format")
  w25 = u16 3 items=["    RS2_STREAM_ANY,", "    RS2_STREAM_DEPTH                            , /**< Native stream of depth data produced by RealSense device */", "    RS2_STREAM_COLOR                            , /**< Native stream of color data captured by RealSense device */", "    RS2_STREAM_INFRARED                         , /**< Native stream of infrared data captured by RealSense device */", "    RS2_STREAM_FISHEYE                          , /**< Native stream of fish-eye (wide) data captured from the dedicate motion camera */", "    RS2_STREAM_GYRO                             , /**< Native stream of gyroscope motion data produced by RealSense device */", "    RS2_STREAM_ACCEL                            , /**< Native stream of accelerometer motion data produced by RealSense device */", "    RS2_STREAM_GPIO                             , /**< Signals from external device connected through GPIO */", "    RS2_STREAM_COUNT"] ("RS Stream")
  w29 = u16 10 items=["    RS2_FORMAT_ANY             , /**< When passed to enable stream, librealsense will try to provide best suited format */", "    RS2_FORMAT_Z16             , /**< 16-bit linear depth values. The depth is meters is equal to depth scale * pixel value. */", "    RS2_FORMAT_DISPARITY16     , /**< 16-bit linear disparity values. The depth in meters is equal to depth scale / pixel value. */", "    RS2_FORMAT_XYZ32F          , /**< 32-bit floating point 3D coordinates. */", "    RS2_FORMAT_YUYV            , /**< Standard YUV pixel format as described in https://en.wikipedia.org/wiki/YUV */", "    RS2_FORMAT_RGB8            , /**< 8-bit red, green and blue channels */", "    RS2_FORMAT_BGR8            , /**< 8-bit blue, green, and red channels -- suitable for OpenCV */", "    RS2_FORMAT_RGBA8           , /**< 8-bit red, green and blue channels + constant alpha channel equal to FF */", "    RS2_FORMAT_BGRA8           , /**< 8-bit blue, green, and red channels + constant alpha channel equal to FF */", "    RS2_FORMAT_Y8              , /**< 8-bit per-pixel grayscale image */", "    RS2_FORMAT_Y16             , /**< 16-bit per-pixel grayscale image */", "    RS2_FORMAT_RAW10           , /**< Four 10-bit luminance values encoded into a 5-byte macropixel */", "    RS2_FORMAT_RAW16           , /**< 16-bit raw image */", "    RS2_FORMAT_RAW8            , /**< 8-bit raw image */", "    RS2_FORMAT_UYVY            , /**< Similar to the standard YUYV pixel format, but packed in a different order */", "    RS2_FORMAT_MOTION_RAW      , /**< Raw data from the motion sensor */", "    RS2_FORMAT_MOTION_XYZ32F   , /**< Motion data packed as 3 32-bit float values, for X, Y, and Z axis */", "    RS2_FORMAT_GPIO_RAW        , /**< Raw data from the external sensors hooked to one of the GPIO's */", "    RS2_FORMAT_COUNT             /**< Number of enumeration values. Not a valid input: intended to be used in for-loops. */"] ("RS Format")
  w28 = u16 3 items=["    RS2_STREAM_ANY,", "    RS2_STREAM_DEPTH                            , /**< Native stream of depth data produced by RealSense device */", "    RS2_STREAM_COLOR                            , /**< Native stream of color data captured by RealSense device */", "    RS2_STREAM_INFRARED                         , /**< Native stream of infrared data captured by RealSense device */", "    RS2_STREAM_FISHEYE                          , /**< Native stream of fish-eye (wide) data captured from the dedicate motion camera */", "    RS2_STREAM_GYRO                             , /**< Native stream of gyroscope motion data produced by RealSense device */", "    RS2_STREAM_ACCEL                            , /**< Native stream of accelerometer motion data produced by RealSense device */", "    RS2_STREAM_GPIO                             , /**< Signals from external device connected through GPIO */", "    RS2_STREAM_COUNT"] ("RS Stream")
  w39 = u16 3 items=["    RS2_STREAM_ANY,", "    RS2_STREAM_DEPTH                            , /**< Native stream of depth data produced by RealSense device */", "    RS2_STREAM_COLOR                            , /**< Native stream of color data captured by RealSense device */", "    RS2_STREAM_INFRARED                         , /**< Native stream of infrared data captured by RealSense device */", "    RS2_STREAM_FISHEYE                          , /**< Native stream of fish-eye (wide) data captured from the dedicate motion camera */", "    RS2_STREAM_GYRO                             , /**< Native stream of gyroscope motion data produced by RealSense device */", "    RS2_STREAM_ACCEL                            , /**< Native stream of accelerometer motion data produced by RealSense device */", "    RS2_STREAM_GPIO                             , /**< Signals from external device connected through GPIO */", "    RS2_STREAM_COUNT"] ("RS Stream")
  w38 = u16 9 items=["    RS2_FORMAT_ANY             , /**< When passed to enable stream, librealsense will try to provide best suited format */", "    RS2_FORMAT_Z16             , /**< 16-bit linear depth values. The depth is meters is equal to depth scale * pixel value. */", "    RS2_FORMAT_DISPARITY16     , /**< 16-bit linear disparity values. The depth in meters is equal to depth scale / pixel value. */", "    RS2_FORMAT_XYZ32F          , /**< 32-bit floating point 3D coordinates. */", "    RS2_FORMAT_YUYV            , /**< Standard YUV pixel format as described in https://en.wikipedia.org/wiki/YUV */", "    RS2_FORMAT_RGB8            , /**< 8-bit red, green and blue channels */", "    RS2_FORMAT_BGR8            , /**< 8-bit blue, green, and red channels -- suitable for OpenCV */", "    RS2_FORMAT_RGBA8           , /**< 8-bit red, green and blue channels + constant alpha channel equal to FF */", "    RS2_FORMAT_BGRA8           , /**< 8-bit blue, green, and red channels + constant alpha channel equal to FF */", "    RS2_FORMAT_Y8              , /**< 8-bit per-pixel grayscale image */", "    RS2_FORMAT_Y16             , /**< 16-bit per-pixel grayscale image */", "    RS2_FORMAT_RAW10           , /**< Four 10-bit luminance values encoded into a 5-byte macropixel */", "    RS2_FORMAT_RAW16           , /**< 16-bit raw image */", "    RS2_FORMAT_RAW8            , /**< 8-bit raw image */", "    RS2_FORMAT_UYVY            , /**< Similar to the standard YUYV pixel format, but packed in a different order */", "    RS2_FORMAT_MOTION_RAW      , /**< Raw data from the motion sensor */", "    RS2_FORMAT_MOTION_XYZ32F   , /**< Motion data packed as 3 32-bit float values, for X, Y, and Z axis */", "    RS2_FORMAT_GPIO_RAW        , /**< Raw data from the external sensors hooked to one of the GPIO's */", "    RS2_FORMAT_COUNT             /**< Number of enumeration values. Not a valid input: intended to be used in for-loops. */"] ("RS Format")
  w40 = u16 3 items=["    RS2_STREAM_ANY,", "    RS2_STREAM_DEPTH                            , /**< Native stream of depth data produced by RealSense device */", "    RS2_STREAM_COLOR                            , /**< Native stream of color data captured by RealSense device */", "    RS2_STREAM_INFRARED                         , /**< Native stream of infrared data captured by RealSense device */", "    RS2_STREAM_FISHEYE                          , /**< Native stream of fish-eye (wide) data captured from the dedicate motion camera */", "    RS2_STREAM_GYRO                             , /**< Native stream of gyroscope motion data produced by RealSense device */", "    RS2_STREAM_ACCEL                            , /**< Native stream of accelerometer motion data produced by RealSense device */", "    RS2_STREAM_GPIO                             , /**< Signals from external device connected through GPIO */", "    RS2_STREAM_COUNT"] ("RS Stream")
  w41 = u16 9 items=["    RS2_FORMAT_ANY             , /**< When passed to enable stream, librealsense will try to provide best suited format */", "    RS2_FORMAT_Z16             , /**< 16-bit linear depth values. The depth is meters is equal to depth scale * pixel value. */", "    RS2_FORMAT_DISPARITY16     , /**< 16-bit linear disparity values. The depth in meters is equal to depth scale / pixel value. */", "    RS2_FORMAT_XYZ32F          , /**< 32-bit floating point 3D coordinates. */", "    RS2_FORMAT_YUYV            , /**< Standard YUV pixel format as described in https://en.wikipedia.org/wiki/YUV */", "    RS2_FORMAT_RGB8            , /**< 8-bit red, green and blue channels */", "    RS2_FORMAT_BGR8            , /**< 8-bit blue, green, and red channels -- suitable for OpenCV */", "    RS2_FORMAT_RGBA8           , /**< 8-bit red, green and blue channels + constant alpha channel equal to FF */", "    RS2_FORMAT_BGRA8           , /**< 8-bit blue, green, and red channels + constant alpha channel equal to FF */", "    RS2_FORMAT_Y8              , /**< 8-bit per-pixel grayscale image */", "    RS2_FORMAT_Y16             , /**< 16-bit per-pixel grayscale image */", "    RS2_FORMAT_RAW10           , /**< Four 10-bit luminance values encoded into a 5-byte macropixel */", "    RS2_FORMAT_RAW16           , /**< 16-bit raw image */", "    RS2_FORMAT_RAW8            , /**< 8-bit raw image */", "    RS2_FORMAT_UYVY            , /**< Similar to the standard YUYV pixel format, but packed in a different order */", "    RS2_FORMAT_MOTION_RAW      , /**< Raw data from the motion sensor */", "    RS2_FORMAT_MOTION_XYZ32F   , /**< Motion data packed as 3 32-bit float values, for X, Y, and Z axis */", "    RS2_FORMAT_GPIO_RAW        , /**< Raw data from the external sensors hooked to one of the GPIO's */", "    RS2_FORMAT_COUNT             /**< Number of enumeration values. Not a valid input: intended to be used in for-loops. */"] ("RS Format")
  w9 = T1 [] ("appended array")
  w52 = u16 3 items=["    RS2_STREAM_ANY,", "    RS2_STREAM_DEPTH                            , /**< Native stream of depth data produced by RealSense device */", "    RS2_STREAM_COLOR                            , /**< Native stream of color data captured by RealSense device */", "    RS2_STREAM_INFRARED                         , /**< Native stream of infrared data captured by RealSense device */", "    RS2_STREAM_FISHEYE                          , /**< Native stream of fish-eye (wide) data captured from the dedicate motion camera */", "    RS2_STREAM_GYRO                             , /**< Native stream of gyroscope motion data produced by RealSense device */", "    RS2_STREAM_ACCEL                            , /**< Native stream of accelerometer motion data produced by RealSense device */", "    RS2_STREAM_GPIO                             , /**< Signals from external device connected through GPIO */", "    RS2_STREAM_COUNT"] ("RS Stream")
  w51 = u16 5 items=["    RS2_FORMAT_ANY             , /**< When passed to enable stream, librealsense will try to provide best suited format */", "    RS2_FORMAT_Z16             , /**< 16-bit linear depth values. The depth is meters is equal to depth scale * pixel value. */", "    RS2_FORMAT_DISPARITY16     , /**< 16-bit linear disparity values. The depth in meters is equal to depth scale / pixel value. */", "    RS2_FORMAT_XYZ32F          , /**< 32-bit floating point 3D coordinates. */", "    RS2_FORMAT_YUYV            , /**< Standard YUV pixel format as described in https://en.wikipedia.org/wiki/YUV */", "    RS2_FORMAT_RGB8            , /**< 8-bit red, green and blue channels */", "    RS2_FORMAT_BGR8            , /**< 8-bit blue, green, and red channels -- suitable for OpenCV */", "    RS2_FORMAT_RGBA8           , /**< 8-bit red, green and blue channels + constant alpha channel equal to FF */", "    RS2_FORMAT_BGRA8           , /**< 8-bit blue, green, and red channels + constant alpha channel equal to FF */", "    RS2_FORMAT_Y8              , /**< 8-bit per-pixel grayscale image */", "    RS2_FORMAT_Y16             , /**< 16-bit per-pixel grayscale image */", "    RS2_FORMAT_RAW10           , /**< Four 10-bit luminance values encoded into a 5-byte macropixel */", "    RS2_FORMAT_RAW16           , /**< 16-bit raw image */", "    RS2_FORMAT_RAW8            , /**< 8-bit raw image */", "    RS2_FORMAT_UYVY            , /**< Similar to the standard YUYV pixel format, but packed in a different order */", "    RS2_FORMAT_MOTION_RAW      , /**< Raw data from the motion sensor */", "    RS2_FORMAT_MOTION_XYZ32F   , /**< Motion data packed as 3 32-bit float values, for X, Y, and Z axis */", "    RS2_FORMAT_GPIO_RAW        , /**< Raw data from the external sensors hooked to one of the GPIO's */", "    RS2_FORMAT_COUNT             /**< Number of enumeration values. Not a valid input: intended to be used in for-loops. */"] ("RS Format")
  w56 = u16 1 items=["    RS2_FORMAT_ANY             , /**< When passed to enable stream, librealsense will try to provide best suited format */", "    RS2_FORMAT_Z16             , /**< 16-bit linear depth values. The depth is meters is equal to depth scale * pixel value. */", "    RS2_FORMAT_DISPARITY16     , /**< 16-bit linear disparity values. The depth in meters is equal to depth scale / pixel value. */", "    RS2_FORMAT_XYZ32F          , /**< 32-bit floating point 3D coordinates. */", "    RS2_FORMAT_YUYV            , /**< Standard YUV pixel format as described in https://en.wikipedia.org/wiki/YUV */", "    RS2_FORMAT_RGB8            , /**< 8-bit red, green and blue channels */", "    RS2_FORMAT_BGR8            , /**< 8-bit blue, green, and red channels -- suitable for OpenCV */", "    RS2_FORMAT_RGBA8           , /**< 8-bit red, green and blue channels + constant alpha channel equal to FF */", "    RS2_FORMAT_BGRA8           , /**< 8-bit blue, green, and red channels + constant alpha channel equal to FF */", "    RS2_FORMAT_Y8              , /**< 8-bit per-pixel grayscale image */", "    RS2_FORMAT_Y16             , /**< 16-bit per-pixel grayscale image */", "    RS2_FORMAT_RAW10           , /**< Four 10-bit luminance values encoded into a 5-byte macropixel */", "    RS2_FORMAT_RAW16           , /**< 16-bit raw image */", "    RS2_FORMAT_RAW8            , /**< 8-bit raw image */", "    RS2_FORMAT_UYVY            , /**< Similar to the standard YUYV pixel format, but packed in a different order */", "    RS2_FORMAT_MOTION_RAW      , /**< Raw data from the motion sensor */", "    RS2_FORMAT_MOTION_XYZ32F   , /**< Motion data packed as 3 32-bit float values, for X, Y, and Z axis */", "    RS2_FORMAT_GPIO_RAW        , /**< Raw data from the external sensors hooked to one of the GPIO's */", "    RS2_FORMAT_COUNT             /**< Number of enumeration values. Not a valid input: intended to be used in for-loops. */"] ("RS Format")
  w57 = u16 1 items=["    RS2_STREAM_ANY,", "    RS2_STREAM_DEPTH                            , /**< Native stream of depth data produced by RealSense device */", "    RS2_STREAM_COLOR                            , /**< Native stream of color data captured by RealSense device */", "    RS2_STREAM_INFRARED                         , /**< Native stream of infrared data captured by RealSense device */", "    RS2_STREAM_FISHEYE                          , /**< Native stream of fish-eye (wide) data captured from the dedicate motion camera */", "    RS2_STREAM_GYRO                             , /**< Native stream of gyroscope motion data produced by RealSense device */", "    RS2_STREAM_ACCEL                            , /**< Native stream of accelerometer motion data produced by RealSense device */", "    RS2_STREAM_GPIO                             , /**< Signals from external device connected through GPIO */", "    RS2_STREAM_COUNT"] ("RS Stream")
  n1 = for {
    tunnel: "Stream profile array" -> [w82] mode=indexing
    shift-right: [w77] -> w37
    shift-left: string[] [] -> [w76]
    shift-right: [w75] -> w35
    shift-left: w9 -> [w74]
    tunnel: w39 -> [w72]
    tunnel: w38 -> [w69]
    # "IR (RIGHT)"
    n2 = Unbundle By Name(w82) -> ("height"=w79:i32, "width"=w80:i32, "fps"=w78:i32, "RS Stream"=w73:u16, "RS Format"=w70:u16, "Profile"=w67:u64, "ppx"=w66:sgl, "ppy"=w65:sgl, "fx"=w64:sgl, "fy"=w63:sgl, "model"=w62:u32, "index"=w61:u16)
    n3 = Equal?(x=w70, y=w69) -> (x = y?=w68:bool)
    n4 = Equal?(x=w73, y=w72) -> (x = y?=w71:bool)
    n5 = Equal?(x=w61, y=u16 2) -> (x = y?=w59:bool)
    n6 = Compound Arithmetic op=AND(w68, w71, w59) -> (w81:bool)
    n7 = case shown="True" w81 {
      tunnel: w80 -> [_ w96]
      tunnel: w79 -> [_ w95]
      tunnel: w78 -> [_ w94]
      tunnel: [w84 w98] -> w77
      tunnel: w76 -> [w84 w97]
      tunnel: [w83 w92] -> w75
      tunnel: w74 -> [w83 w91]
      tunnel: w67 -> [_ w90]
      tunnel: w66 -> [_ w89]
      tunnel: w65 -> [_ w88]
      tunnel: w64 -> [_ w87]
      tunnel: w63 -> [_ w86]
      tunnel: w62 -> [_ w85]
      frame False {
      }
      frame True {
        n8 = Bundle("width"=w96, "height"=w95, "fps"=w94, "Profile"=w90, "ppx"=w89, "ppy"=w88, "fx"=w87, "fy"=w86, "model"=w85) -> (w93:T3)  [unwired: 1 in]
        n9 = Build Array (concatenate)(w91, w93) -> (w92:T1)
        n10 = Format Into String(format string="%d x %d @%dfps", w96, w95, w94) -> (resulting string=w99:string)  [unwired: 2 in, 1 out]
        n11 = Build Array (concatenate)(w97, w99) -> (w98:string[])
      }
    }
  }
  n12 = for {
    tunnel: "Stream profile array" -> [w124] mode=indexing
    shift-right: [w119] -> w42
    shift-left: string[] [] -> [w118]
    shift-right: [w117] -> w44
    shift-left: w9 -> [w116]
    tunnel: w40 -> [w114]
    tunnel: w41 -> [w111]
    # "IR (LEFT)"
    n13 = Unbundle By Name(w124) -> ("height"=w121:i32, "width"=w122:i32, "fps"=w120:i32, "RS Stream"=w115:u16, "RS Format"=w112:u16, "Profile"=w110:u64, "ppx"=w109:sgl, "ppy"=w108:sgl, "fx"=w107:sgl, "fy"=w106:sgl, "model"=w105:u32, "index"=w103:u16)
    n14 = Equal?(x=w112, y=w111) -> (x = y?=w104:bool)
    n15 = Equal?(x=w115, y=w114) -> (x = y?=w113:bool)
    n16 = Equal?(x=u16 1, y=w103) -> (x = y?=w101:bool)
    n17 = Compound Arithmetic op=AND(w104, w113, w101) -> (w123:bool)
    n18 = case shown="True" w123 {
      tunnel: w122 -> [_ w138]
      tunnel: w121 -> [_ w137]
      tunnel: w120 -> [_ w136]
      tunnel: [w126 w140] -> w119
      tunnel: w118 -> [w126 w139]
      tunnel: [w125 w134] -> w117
      tunnel: w116 -> [w125 w133]
      tunnel: w110 -> [_ w132]
      tunnel: w109 -> [_ w131]
      tunnel: w108 -> [_ w130]
      tunnel: w107 -> [_ w129]
      tunnel: w106 -> [_ w128]
      tunnel: w105 -> [_ w127]
      frame False {
      }
      frame True {
        n19 = Bundle("width"=w138, "height"=w137, "fps"=w136, "Profile"=w132, "ppx"=w131, "ppy"=w130, "fx"=w129, "fy"=w128, "model"=w127) -> (w135:T3)  [unwired: 1 in]
        n20 = Build Array (concatenate)(w133, w135) -> (w134:T1)
        n21 = Format Into String(format string="%d x %d @%dfps", w138, w137, w136) -> (resulting string=w141:string)  [unwired: 2 in, 1 out]
        n22 = Build Array (concatenate)(w139, w141) -> (w140:string[])
      }
    }
  }
  n23 = for {
    tunnel: "Stream profile array" -> [w166] mode=indexing
    shift-right: [w161] -> w50
    shift-left: string[] [] -> [w160]
    shift-right: [w159] -> w48
    shift-left: w9 -> [w158]
    tunnel: w52 -> [w156]
    tunnel: w51 -> [w153]
    # "COLOR (LEFT)"
    n24 = Unbundle By Name(w166) -> ("height"=w163:i32, "width"=w164:i32, "fps"=w162:i32, "RS Stream"=w157:u16, "RS Format"=w154:u16, "Profile"=w151:u64, "ppx"=w150:sgl, "ppy"=w149:sgl, "fx"=w148:sgl, "fy"=w147:sgl, "model"=w146:u32, "index"=w145:u16)
    n25 = Equal?(x=w154, y=w153) -> (x = y?=w152:bool)
    n26 = Equal?(x=w157, y=w156) -> (x = y?=w155:bool)
    n27 = Equal?(x=w145, y=u16 0) -> (x = y?=w143:bool)
    n28 = Compound Arithmetic op=AND(w152, w155, w143) -> (w165:bool)
    n29 = case shown="True" w165 {
      tunnel: w164 -> [_ w180]
      tunnel: w163 -> [_ w179]
      tunnel: w162 -> [_ w178]
      tunnel: [w168 w182] -> w161
      tunnel: w160 -> [w168 w181]
      tunnel: [w167 w176] -> w159
      tunnel: w158 -> [w167 w175]
      tunnel: w151 -> [_ w174]
      tunnel: w150 -> [_ w173]
      tunnel: w149 -> [_ w172]
      tunnel: w148 -> [_ w171]
      tunnel: w147 -> [_ w170]
      tunnel: w146 -> [_ w169]
      frame False {
      }
      frame True {
        n30 = Bundle("width"=w180, "height"=w179, "fps"=w178, "Profile"=w174, "ppx"=w173, "ppy"=w172, "fx"=w171, "fy"=w170, "model"=w169) -> (w177:T3)  [unwired: 1 in]
        n31 = Build Array (concatenate)(w175, w177) -> (w176:T1)
        n32 = Format Into String(format string="%d x %d @%dfps", w180, w179, w178) -> (resulting string=w183:string)  [unwired: 2 in, 1 out]
        n33 = Build Array (concatenate)(w181, w183) -> (w182:string[])
      }
    }
  }
  n34 = for {
    tunnel: "Stream profile array" -> [w208] mode=indexing
    shift-right: [w203] -> w55
    shift-left: string[] [] -> [w202]
    shift-right: [w201] -> w53
    shift-left: w9 -> [w200]
    tunnel: w57 -> [w198]
    tunnel: w56 -> [w195]
    # "DEPTH"
    n35 = Unbundle By Name(w208) -> ("height"=w205:i32, "width"=w206:i32, "fps"=w204:i32, "RS Stream"=w199:u16, "RS Format"=w196:u16, "Profile"=w193:u64, "ppx"=w192:sgl, "ppy"=w191:sgl, "fx"=w190:sgl, "fy"=w189:sgl, "model"=w188:u32, "index"=w187:u16)
    n36 = Equal?(x=w196, y=w195) -> (x = y?=w194:bool)
    n37 = Equal?(x=w199, y=w198) -> (x = y?=w197:bool)
    n38 = Equal?(x=w187, y=u16 0) -> (x = y?=w185:bool)
    n39 = Compound Arithmetic op=AND(w194, w197, w185) -> (w207:bool)
    n40 = case shown="True" w207 {
      tunnel: w206 -> [_ w222]
      tunnel: w205 -> [_ w221]
      tunnel: w204 -> [_ w220]
      tunnel: [w210 w224] -> w203
      tunnel: w202 -> [w210 w223]
      tunnel: [w209 w219] -> w201
      tunnel: w200 -> [w209 w211]
      tunnel: w193 -> [_ w218]
      tunnel: w192 -> [_ w217]
      tunnel: w191 -> [_ w216]
      tunnel: w190 -> [_ w215]
      tunnel: w189 -> [_ w214]
      tunnel: w188 -> [_ w213]
      frame False {
      }
      frame True {
        n41 = Bundle("width"=w222, "height"=w221, "fps"=w220, "Profile"=w218, "ppx"=w217, "ppy"=w216, "fx"=w215, "fy"=w214, "model"=w213) -> (w212:T3)  [unwired: 1 in]
        n42 = Build Array (concatenate)(w211, w212) -> (w219:T1)
        n43 = Format Into String(format string="%d x %d @%dfps", w222, w221, w220) -> (resulting string=w225:string)  [unwired: 2 in, 1 out]
        n44 = Build Array (concatenate)(w223, w225) -> (w224:string[])
      }
    }
  }
  n45 = for {
    tunnel: "Stream profile array" -> [w249] mode=indexing
    shift-right: [w244] -> w30
    shift-left: string[] [] -> [w243]
    shift-right: [w242] -> w32
    shift-left: w9 -> [w241]
    tunnel: w28 -> [w239]
    tunnel: w29 -> [_]
    # "Unrectified L"
    n46 = Unbundle By Name(w249) -> ("height"=w246:i32, "width"=w247:i32, "fps"=w245:i32, "RS Stream"=w240:u16, "Profile"=w237:u64, "ppx"=w231:sgl, "ppy"=w236:sgl, "fx"=w235:sgl, "fy"=w234:sgl, "model"=w230:u32, "index"=w228:u16)  [unwired: 1 out]
    n47 = Equal?(x=w240, y=w239) -> (x = y?=w238:bool)
    n48 = Equal?(x=w230, y=u16 0) -> (x = y?=w232:bool)
    n49 = Equal?(x=w228, y=u16 1) -> (x = y?=w227:bool)
    n50 = Compound Arithmetic op=AND(w238, w232, w227) -> (w248:bool)
    n51 = case shown="True" w248 {
      tunnel: w247 -> [_ w263]
      tunnel: w246 -> [_ w262]
      tunnel: w245 -> [_ w261]
      tunnel: [w251 w265] -> w244
      tunnel: w243 -> [w251 w264]
      tunnel: [w250 w260] -> w242
      tunnel: w241 -> [w250 w252]
      tunnel: w237 -> [_ w259]
      tunnel: w231 -> [_ w258]
      tunnel: w236 -> [_ w257]
      tunnel: w235 -> [_ w256]
      tunnel: w234 -> [_ w255]
      tunnel: w230 -> [_ w254]
      frame False {
      }
      frame True {
        n52 = Bundle("width"=w263, "height"=w262, "fps"=w261, "Profile"=w259, "ppx"=w258, "ppy"=w257, "fx"=w256, "fy"=w255, "model"=w254) -> (w253:T3)  [unwired: 1 in]
        n53 = Build Array (concatenate)(w252, w253) -> (w260:T1)
        n54 = Format Into String(format string="%d x %d @%dfps", w263, w262, w261) -> (resulting string=w266:string)  [unwired: 2 in, 1 out]
        n55 = Build Array (concatenate)(w264, w266) -> (w265:string[])
      }
    }
  }
  n56 = for {
    tunnel: "Stream profile array" -> [w290] mode=indexing
    shift-right: [w285] -> w23
    shift-left: string[] [] -> [w284]
    shift-right: [w283] -> w21
    shift-left: w9 -> [w282]
    tunnel: w25 -> [w280]
    tunnel: w24 -> [_]
    # "Unrectified L"
    n57 = Unbundle By Name(w290) -> ("height"=w287:i32, "width"=w288:i32, "fps"=w286:i32, "RS Stream"=w281:u16, "Profile"=w278:u64, "ppx"=w272:sgl, "ppy"=w277:sgl, "fx"=w276:sgl, "fy"=w275:sgl, "model"=w271:u32, "index"=w269:u16)  [unwired: 1 out]
    n58 = Equal?(x=w281, y=w280) -> (x = y?=w279:bool)
    n59 = Equal?(x=w271, y=u16 0) -> (x = y?=w273:bool)
    n60 = Equal?(x=w269, y=u16 2) -> (x = y?=w268:bool)
    n61 = Compound Arithmetic op=AND(w279, w273, w268) -> (w289:bool)
    n62 = case shown="True" w289 {
      tunnel: w288 -> [_ w304]
      tunnel: w287 -> [_ w303]
      tunnel: w286 -> [_ w302]
      tunnel: [w292 w306] -> w285
      tunnel: w284 -> [w292 w305]
      tunnel: [w291 w301] -> w283
      tunnel: w282 -> [w291 w293]
      tunnel: w278 -> [_ w300]
      tunnel: w272 -> [_ w299]
      tunnel: w277 -> [_ w298]
      tunnel: w276 -> [_ w297]
      tunnel: w275 -> [_ w296]
      tunnel: w271 -> [_ w295]
      frame False {
      }
      frame True {
        n63 = Bundle("width"=w304, "height"=w303, "fps"=w302, "Profile"=w300, "ppx"=w299, "ppy"=w298, "fx"=w297, "fy"=w296, "model"=w295) -> (w294:T3)  [unwired: 1 in]
        n64 = Build Array (concatenate)(w293, w294) -> (w301:T1)
        n65 = Format Into String(format string="%d x %d @%dfps", w304, w303, w302) -> (resulting string=w307:string)  [unwired: 2 in, 1 out]
        n66 = Build Array (concatenate)(w305, w307) -> (w306:string[])
      }
    }
  }
  n67 = for {
    tunnel: "Stream profile array" -> [w332] mode=indexing
    shift-right: [w327] -> w13
    shift-left: string[] [] -> [w326]
    shift-right: [w325] -> w15
    shift-left: w9 -> [w324]
    tunnel: w11 -> [w322]
    tunnel: w12 -> [w310]
    # "External RGB"
    n68 = Unbundle By Name(w332) -> ("height"=w329:i32, "width"=w330:i32, "fps"=w328:i32, "RS Stream"=w323:u16, "RS Format"=w311:u16, "Profile"=w320:u64, "ppx"=w316:sgl, "ppy"=w319:sgl, "fx"=w318:sgl, "fy"=w317:sgl, "model"=w315:u32, "index"=w313:u16)
    n69 = Equal?(x=w323, y=w322) -> (x = y?=w321:bool)
    n70 = Equal?(x=w313, y=u16 0) -> (x = y?=w312:bool)
    n71 = Equal?(x=w311, y=w310) -> (x = y?=w309:bool)
    n72 = Compound Arithmetic op=AND(w321, w312, w309) -> (w331:bool)
    n73 = case shown="True" w331 {
      tunnel: w330 -> [_ w346]
      tunnel: w329 -> [_ w345]
      tunnel: w328 -> [_ w344]
      tunnel: [w334 w348] -> w327
      tunnel: w326 -> [w334 w347]
      tunnel: [w333 w343] -> w325
      tunnel: w324 -> [w333 w335]
      tunnel: w320 -> [_ w342]
      tunnel: w316 -> [_ w341]
      tunnel: w319 -> [_ w340]
      tunnel: w318 -> [_ w339]
      tunnel: w317 -> [_ w338]
      tunnel: w315 -> [_ w337]
      frame False {
      }
      frame True {
        n74 = Bundle("width"=w346, "height"=w345, "fps"=w344, "Profile"=w342, "ppx"=w341, "ppy"=w340, "fx"=w339, "fy"=w338, "model"=w337) -> (w336:T3)  [unwired: 1 in]
        n75 = Build Array (concatenate)(w335, w336) -> (w343:T1)
        n76 = Format Into String(format string="%d x %d @%dfps", w346, w345, w344) -> (resulting string=w349:string)  [unwired: 2 in, 1 out]
        n77 = Build Array (concatenate)(w347, w349) -> (w348:string[])
      }
    }
  }
  n78 = for {
    tunnel: "Stream profile array" -> [w374] mode=indexing
    shift-right: [w369] -> w5
    shift-left: string[] [] -> [w368]
    shift-right: [w367] -> w7
    shift-left: _ -> [w366]
    tunnel: w1 -> [w364]
    tunnel: u16 20 ("RS Format") -> [w361]
    # "DEPTH compressed"
    n79 = Unbundle By Name(w374) -> ("height"=w371:i32, "width"=w372:i32, "fps"=w370:i32, "RS Stream"=w365:u16, "RS Format"=w362:u16, "Profile"=w359:u64, "ppx"=w358:sgl, "ppy"=w357:sgl, "fx"=w356:sgl, "fy"=w355:sgl, "model"=w354:u32, "index"=w353:u16)
    n80 = Equal?(x=w362, y=w361) -> (x = y?=w360:bool)
    n81 = Equal?(x=w365, y=w364) -> (x = y?=w363:bool)
    n82 = Equal?(x=w353, y=u16 0) -> (x = y?=w351:bool)
    n83 = Compound Arithmetic op=AND(w360, w363, w351) -> (w373:bool)
    n84 = case shown="True" w373 {
      tunnel: w372 -> [_ w388]
      tunnel: w371 -> [_ w387]
      tunnel: w370 -> [_ w386]
      tunnel: [w376 w390] -> w369
      tunnel: w368 -> [w376 w389]
      tunnel: [w375 w385] -> w367
      tunnel: w366 -> [w375 w377]
      tunnel: w359 -> [_ w384]
      tunnel: w358 -> [_ w383]
      tunnel: w357 -> [_ w382]
      tunnel: w356 -> [_ w381]
      tunnel: w355 -> [_ w380]
      tunnel: w354 -> [_ w379]
      frame False {
      }
      frame True {
        n85 = Bundle("width"=w388, "height"=w387, "fps"=w386, "Profile"=w384, "ppx"=w383, "ppy"=w382, "fx"=w381, "fy"=w380, "model"=w379) -> (w378:T3)  [unwired: 1 in]
        n86 = Build Array (concatenate)(w377, w378) -> (w385:T1)
        n87 = Format Into String(format string="%d x %d @%dfps", w388, w387, w386) -> (resulting string=w391:string)  [unwired: 2 in, 1 out]
        n88 = Build Array (concatenate)(w389, w391) -> (w390:string[])
      }
    }
  }
  n89 = Reverse 1D Array(array=w42) -> (reversed array=→"IR Left Array":string[])
  n90 = Reverse 1D Array(array=w44) -> (reversed array=→"IR left":T1)
  n91 = Reverse 1D Array(array=w53) -> (reversed array=→"Depth Stream":T1)
  n92 = Reverse 1D Array(array=w55) -> (reversed array=→"Depth Stream strings":string[])
  n93 = Reverse 1D Array(array=w32) -> (reversed array=→"Unrectified L IR":T1)
  n94 = Reverse 1D Array(array=w30) -> (reversed array=→"Unrectified L IR":string[])
  n95 = Reverse 1D Array(array=w21) -> (reversed array=→"Unrectified R  IR":T1)
  n96 = Reverse 1D Array(array=w23) -> (reversed array=→"Unrectified R IR":string[])
  n97 = Reverse 1D Array(array=w15) -> (reversed array=→"RGB ext.":T1)
  n98 = Reverse 1D Array(array=w13) -> (reversed array=→"RGB ext.":string[])
  n99 = Reverse 1D Array(array=w7) -> (reversed array=→"Depth Stream Compress.":T1)
  n100 = Reverse 1D Array(array=w5) -> (reversed array=→"Depth Stream strings Compress":string[])
  n101 = Reverse 1D Array(array=w35) -> (reversed array=→"IR Right":T1)
  n102 = Reverse 1D Array(array=w37) -> (reversed array=→"IR Right Array":string[])
  n103 = Reverse 1D Array(array=w48) -> (reversed array=→"Color Left":T1)
  n104 = Reverse 1D Array(array=w50) -> (reversed array=→"Color Left Array":string[])
